vi "FlexMag recipe file.vi"() -> ()   [LabVIEW 2018]
uses:
  <vilib>/Utility/file.llb/Read Delimited Spreadsheet (string).vi
panel:
  in  "redundant":enum32{"Page 1", "Page 2"}(tab)
  in  "dc step length 20":dbl
  in  "dc step length 19":dbl
  in  "dc step length 18":dbl
  in  "dc step length 17":dbl
  in  "dc step length 16":dbl
  in  "dc step length 15":dbl
  in  "dc step length 14":dbl
  in  "dc step length 13":dbl
  in  "dc step length 12":dbl
  in  "dc step length 11":dbl
  in  "dc step length 10":dbl=100.0
  in  "dc step length 9":dbl=100.0
  in  "dc step length 8":dbl=100.0
  in  "dc step length 7":dbl=100.0
  in  "dc step length 6":dbl=100.0
  in  "dc step length 5":dbl=100.0
  in  "dc step length 4":dbl=100.0
  in  "dc step length 3":dbl=100.0
  in  "dc step length 2":dbl=100.0
  in  "dc step length 1":dbl=100.0
  in  "rf step length 20":dbl
  in  "rf step length 19":dbl
  in  "rf step length 18":dbl
  in  "rf step length 17":dbl
  in  "rf step length 16":dbl
  in  "rf step length 15":dbl
  in  "rf step length 14":dbl
  in  "rf step length 13":dbl
  in  "rf step length 12":dbl
  in  "rf step length 11":dbl
  in  "rf step length 1":dbl
  in  "rf step length 2":dbl
  in  "rf step length 3":dbl
  in  "rf step length 4":dbl
  in  "rf step length 5":dbl
  in  "rf step length 6":dbl
  in  "rf step length 7":dbl
  in  "rf step length 8":dbl
  in  "rf step length 9":dbl
  in  "rf step length 10":dbl
  in  "core diameter":dbl=93.0
  in  "left initial diameter":dbl=94.0
  in  "web thickness":dbl=50.0
  out "total length":dbl=500.0
  out "error out 2":errorcluster caption="error out"
  out "error out":errorcluster
  in  "hidden tab":enum32{"Page 1"}(tab)
  out "L dc length step 20":string
  out "L dc length step 19":string
  out "L dc length step 18":string
  out "L dc length step 17":string
  out "L dc length step 16":string
  out "L dc length step 15":string
  out "L dc length step 14":string
  out "L dc length step 13":string
  out "L dc length step 12":string
  out "L dc length step 11":string
  out "L dc power step 20":string
  out "L dc power step 19":string
  out "L dc power step 18":string
  out "L dc power step 17":string
  out "L dc power step 16":string
  out "L dc power step 15":string
  out "L dc power step 14":string
  out "L dc power step 13":string
  out "L dc power step 12":string
  out "L dc power step 11":string
  out "L pressure":string
  out "L argon flow":string
  out "L rf length step 10":string
  out "L rf length step 9":string
  out "L rf length step 8":string
  out "L rf length step 7":string
  out "L rf length step 6":string
  out "L rf length step 5":string
  out "L rf length step 4":string
  out "L rf length step 3":string
  out "L rf length step 2":string
  out "L rf length step 1":string
  out "L rf power step 10":string
  out "L rf power step 9":string
  out "L rf power step 8":string
  out "L rf power step 7":string
  out "L rf power step 6":string
  out "L rf power step 5":string
  out "L rf power step 4":string
  out "L rf power step 3":string
  out "L rf power step 2":string
  out "L rf power step 1":string
  out "L dc length step 10":string
  out "L dc length step 9":string
  out "L dc length step 8":string
  out "L dc length step 7":string
  out "L dc length step 6":string
  out "L dc length step 5":string
  out "L dc length step 4":string
  out "L dc length step 3":string
  out "L dc length step 2":string
  out "L dc length step 1":string
  out "L dc power step 10":string
  out "L dc power step 9":string
  out "L dc power step 8":string
  out "L dc power step 7":string
  out "L dc power step 6":string
  out "L dc power step 5":string
  out "L dc power step 4":string
  out "L dc power step 3":string
  out "L dc power step 2":string
  out "L dc power step 1":string
  out "L microwave power":string
  out "L chamber selection":string
  out "L single process type selection":string
  out "L tension  value":string
  out "L web speed":string
  out "L web thickness":string
  out "L left init diamater":string
  out "L core diamater":string
  out "L web selection":string
  out "L recipe selection":string
  out "L sbs name":string
  out "L recipe name":string
  out "total length error":bool
  out "left diameter after roll":dbl=8.0
  out "done":bool
  out "L dc step number":string
  out "L rf step number":string
  out "L rf length step 11":string
  out "L rf length step 12":string
  out "L rf length step 13":string
  out "L rf length step 14":string
  out "L rf length step 15":string
  out "L rf length step 16":string
  out "L rf length step 17":string
  out "L rf length step 18":string
  out "L rf length step 19":string
  out "L rf length step 20":string
  out "L rf power step 11":string
  out "L rf power step 12":string
  out "L rf power step 13":string
  out "L rf power step 14":string
  out "L rf power step 15":string
  out "L rf power step 16":string
  out "L rf power step 17":string
  out "L rf power step 18":string
  out "L rf power step 19":string
  out "L rf power step 20":string
  in  "steplist tab RF":enum32{"Page 1", "Page 2"}(tab)
  in  "rf step watt 20":dbl
  in  "rf step watt 19":dbl
  in  "rf step watt 18":dbl
  in  "rf step watt 17":dbl
  in  "rf step watt 16":dbl
  in  "rf step watt 15":dbl
  in  "rf step watt 14":dbl
  in  "rf step watt 13":dbl
  in  "rf step watt 12":dbl
  in  "rf step watt 11":dbl
  in  "rf step watt 1":dbl
  in  "rf step watt 2":dbl
  in  "rf step watt 3":dbl
  in  "rf step watt 4":dbl
  in  "rf step watt 7":dbl
  in  "rf step watt 8":dbl
  in  "rf step watt 5":dbl
  in  "rf step watt 6":dbl
  in  "rf step watt 9":dbl
  in  "rf step watt 10":dbl
  in  "Step Number RF":u16(ring) items=["step 1"=1, "step 2"=2, "step 3"=3, "step 4"=4, "step 5"=5, "step 6"=6, "step 7"=7, "step 8"=8, "step 9"=9, "step 10"=10, "step 11"=11, "step 12"=12, "step 13"=13, "step 14"=14, "step 15"=15, "step 16"=16, "step 17"=17, "step 18"=18, "step 19"=19, "step 20"=20]
  out "concatenated string":string
  in  "steplist tab DC":enum32{"Page 1", "Page 2"}(tab)
  in  "dc step watt 1":dbl
  in  "dc step watt 2":dbl
  in  "dc step watt 3":dbl
  in  "dc step watt 4":dbl
  in  "dc step watt 5":dbl
  in  "dc step watt 6":dbl
  in  "dc step watt 7":dbl
  in  "dc step watt 8":dbl
  in  "dc step watt 9":dbl
  in  "dc step watt 10":dbl
  in  "Step Number DC":u16(ring) items=["step 1"=1, "step 2"=2, "step 3"=3, "step 4"=4, "step 5"=5, "step 6"=6, "step 7"=7, "step 8"=8, "step 9"=9, "step 10"=10, "step 11"=11, "step 12"=12, "step 13"=13, "step 14"=14, "step 15"=15, "step 16"=16, "step 17"=17, "step 18"=18, "step 19"=19, "step 20"=20]
  in  "dc step watt 20":dbl
  in  "dc step watt 19":dbl
  in  "dc step watt 18":dbl
  in  "dc step watt 17":dbl
  in  "dc step watt 16":dbl
  in  "dc step watt 15":dbl
  in  "dc step watt 14":dbl
  in  "dc step watt 13":dbl
  in  "dc step watt 12":dbl
  in  "dc step watt 11":dbl
  in  "General tab sub vi":enum32{"Page 1"}(tab)
  in  "Pressure set mbar":dbl=0.007 format="%#_1e"
  in  "Ar set sccm":dbl=40.0
  in  "CANCEL":bool
  in  "SAVE":bool
  in  "web-other tab":T1(tab)
  in  "tension value":dbl=10.0
  in  "web speed":dbl=550.0
  in  "CALCULATE":bool
  in  "Web Selection":u16(ring) items=["web", "other"]
  in  "Recipe Selection":u16(ring) items=["single recipe", "multilayer recipe"]
  in  "Recipe Name":string
  in  "Substrate Material":string
  in  "recipe selection":T2(tab)
  in  "single process selection":enum32{"microwave", "dcsputter", "rfsputter"}(radio)
  in  "single process selection":T3(tab)
  in  "power microwave":dbl
  in  "DC Sputter Chamber Selection":enum32{"chamber II", "chamber III"}(radio)
  in  "power rf":dbl
  in  "web speed ch III ml":dbl=250.0
  in  "web speed ch II ml":dbl=250.0
  in  "LOAD":bool
  in  "SHOW":bool
  in  "password":string
  # "length(cm)"
  # "length(cm)"
  # "Core Diameter"
  # "mm"
  # "Left InitialDiameter"
  # "mm"
  # "µm"
  # "Web Thickness"
  # "cm"
  # "Total Length"
  # "Step List(RF)"
  # "Step Number"
  # "power(watt)"
  # "Step 1"
  # "Step 2"
  # "Step 3"
  # "Step 4"
  # "Step 5"
  # "Step 6"
  # "Step 7"
  # "Step 8"
  # "Step 9"
  # "Step 10"
  # "Step 11"
  # "Step 12"
  # "Step 13"
  # "Step 14"
  # "Step 15"
  # "Step 16"
  # "Step 17"
  # "Step 18"
  # "Step 19"
  # "Step 20"
  # "Step List(DC)"
  # "Stem Number"
  # "power(watt)"
  # "Step 1"
  # "Step 2"
  # "Step 3"
  # "Step 4"
  # "Step 5"
  # "Step 6"
  # "Step 7"
  # "Step 8"
  # "Step 9"
  # "Step 10"
  # "Step 11"
  # "Step 12"
  # "Step 13"
  # "Step 14"
  # "Step 15"
  # "Step 16"
  # "Step 17"
  # "Step 18"
  # "Step 19"
  # "Step 20"
  # "Recipe Name"
  # "Subsrate Material"
  # "Recipe Selection"
  # "Web Selection"
  # "Argon Flow"
  # "sccm"
  # "Set Pressure"
  # "mbar"
  # "Web Speed"
  # "cm/min"
  # "Tension Value"
  # "N"
  # "Power"
  # "watt"
  # "Power"
  # "watt"
  # "DCPS PARAMETERS"
  # "Chamber III"
  # "Chamber II"
  # "Web Speed"
  # "cm/min"
  # "Web Speed"
  # "cm/min"
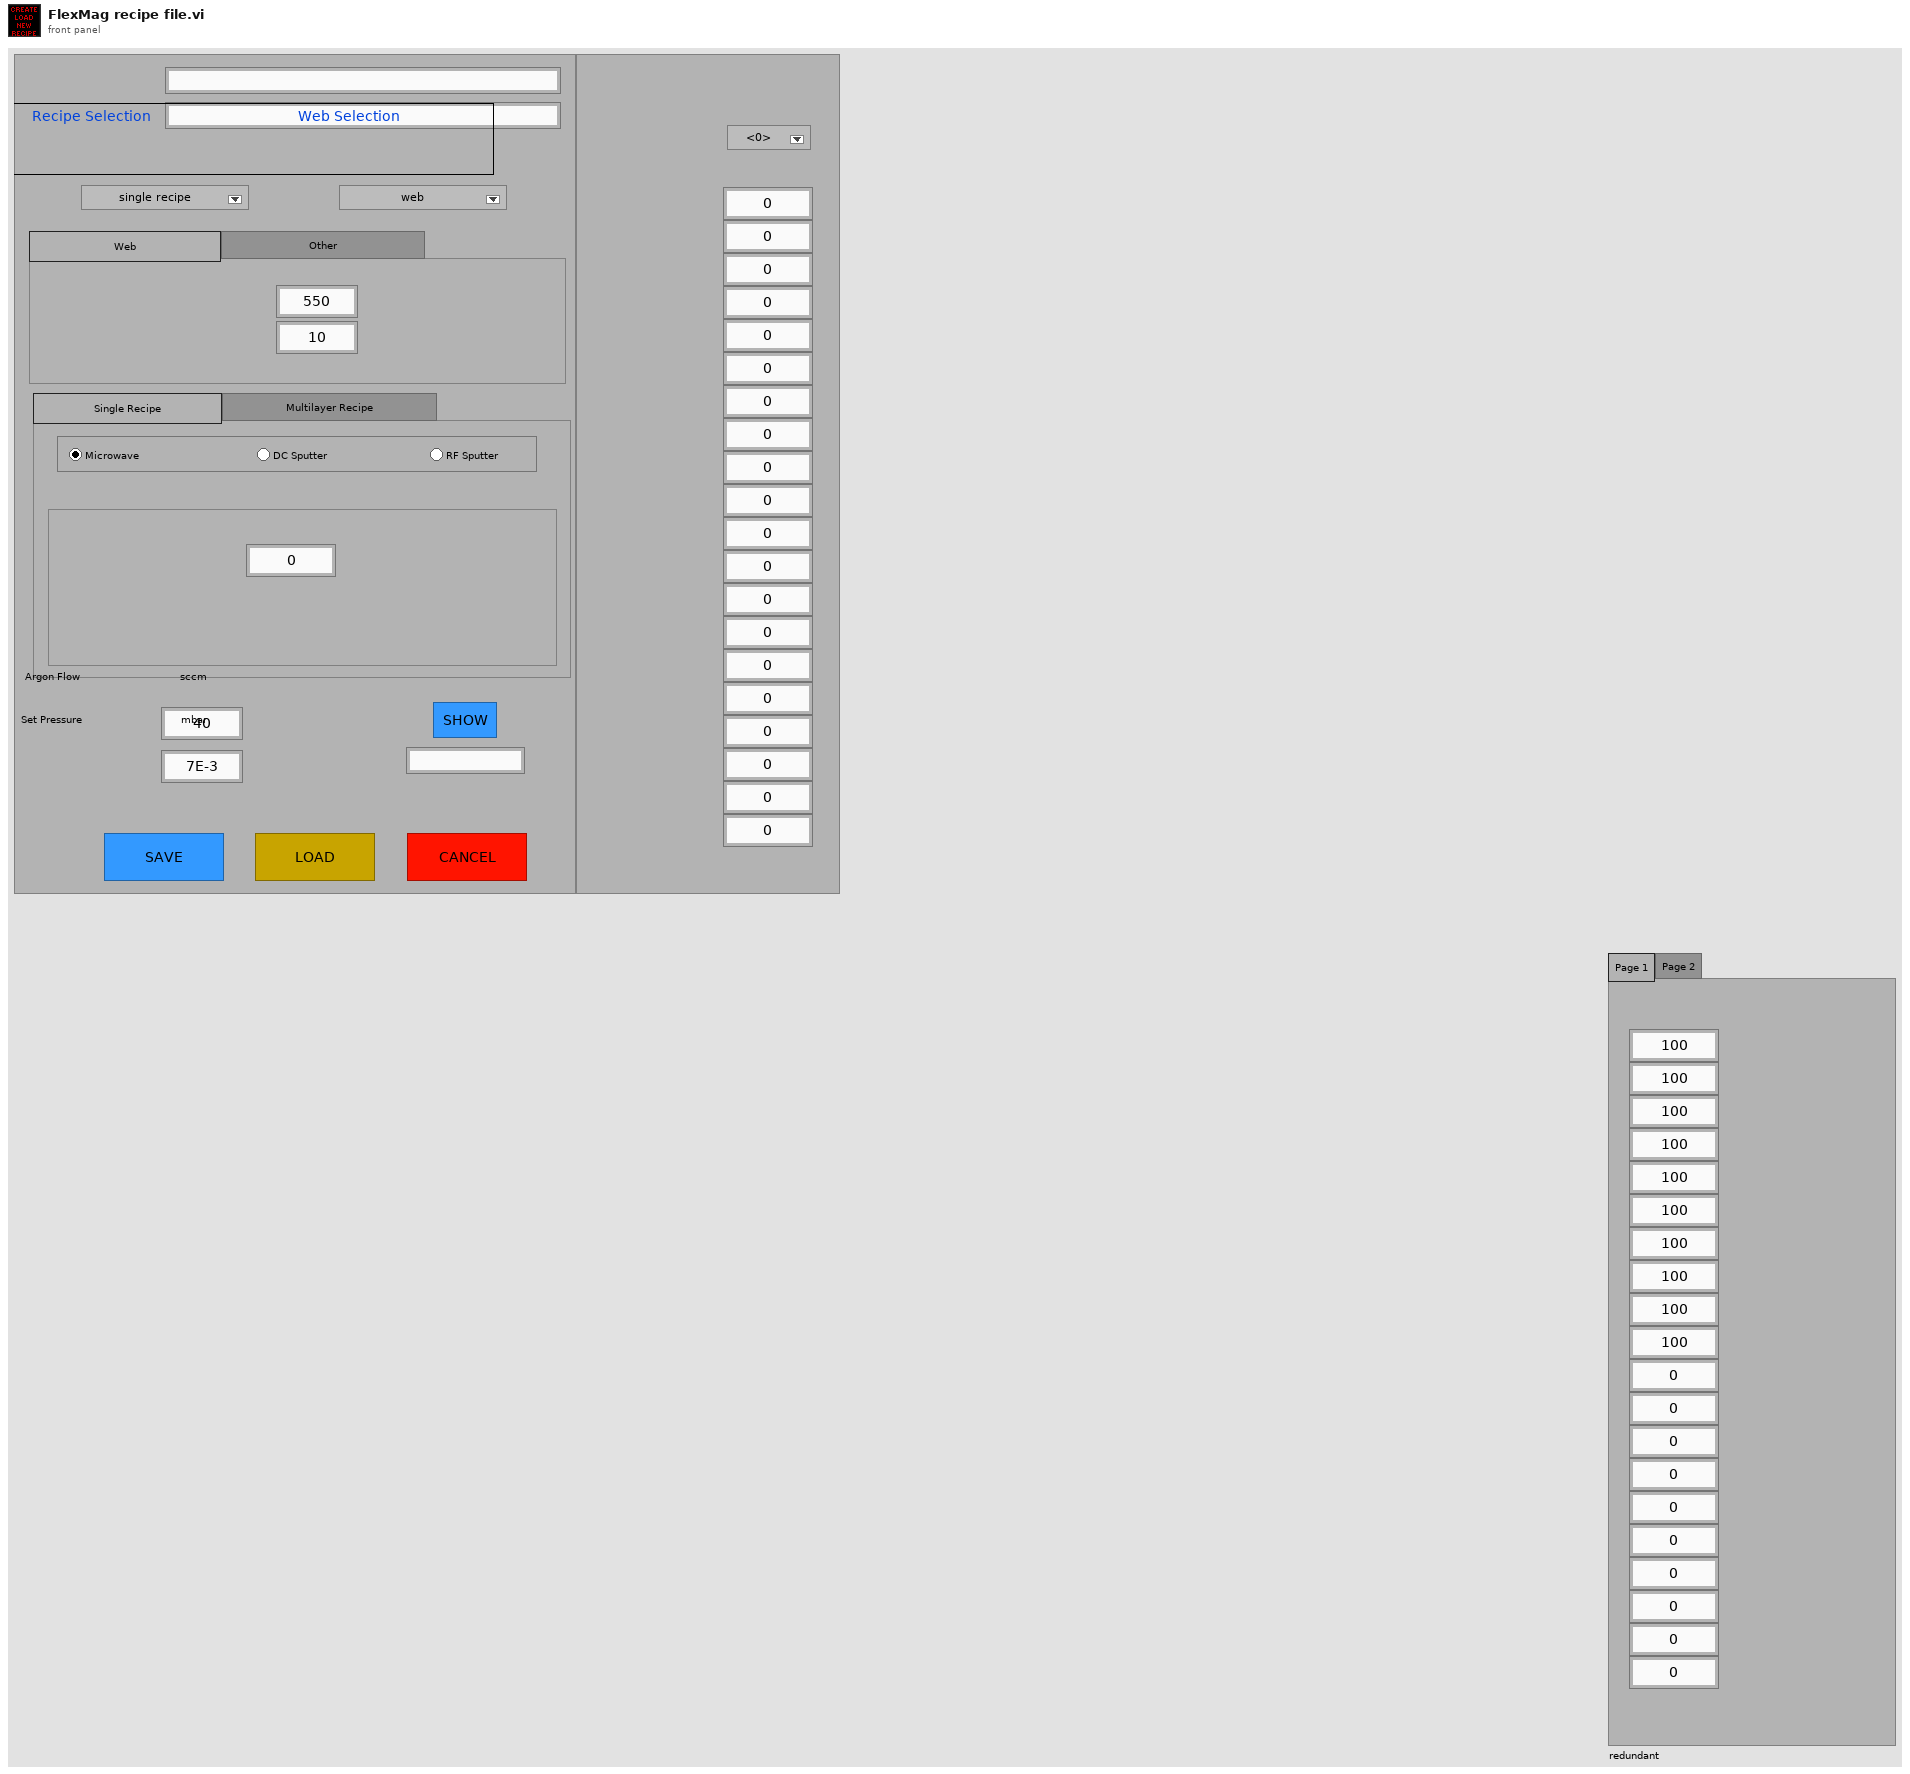
[diagram p1: front panel]
types:
  T1 = enum32{"Web                                                    ", "Other                                                      "}
  T2 = enum32{"Single Recipe                                    ", "Multilayer Recipe                                      "}
  T3 = enum32{"Microwave                ", "DC Sputter                   ", "RF Sputter                         "}
  T4 = enum16{"open", "replace", "create", "open or create", "replace or create", "replace or create with confirmation"}
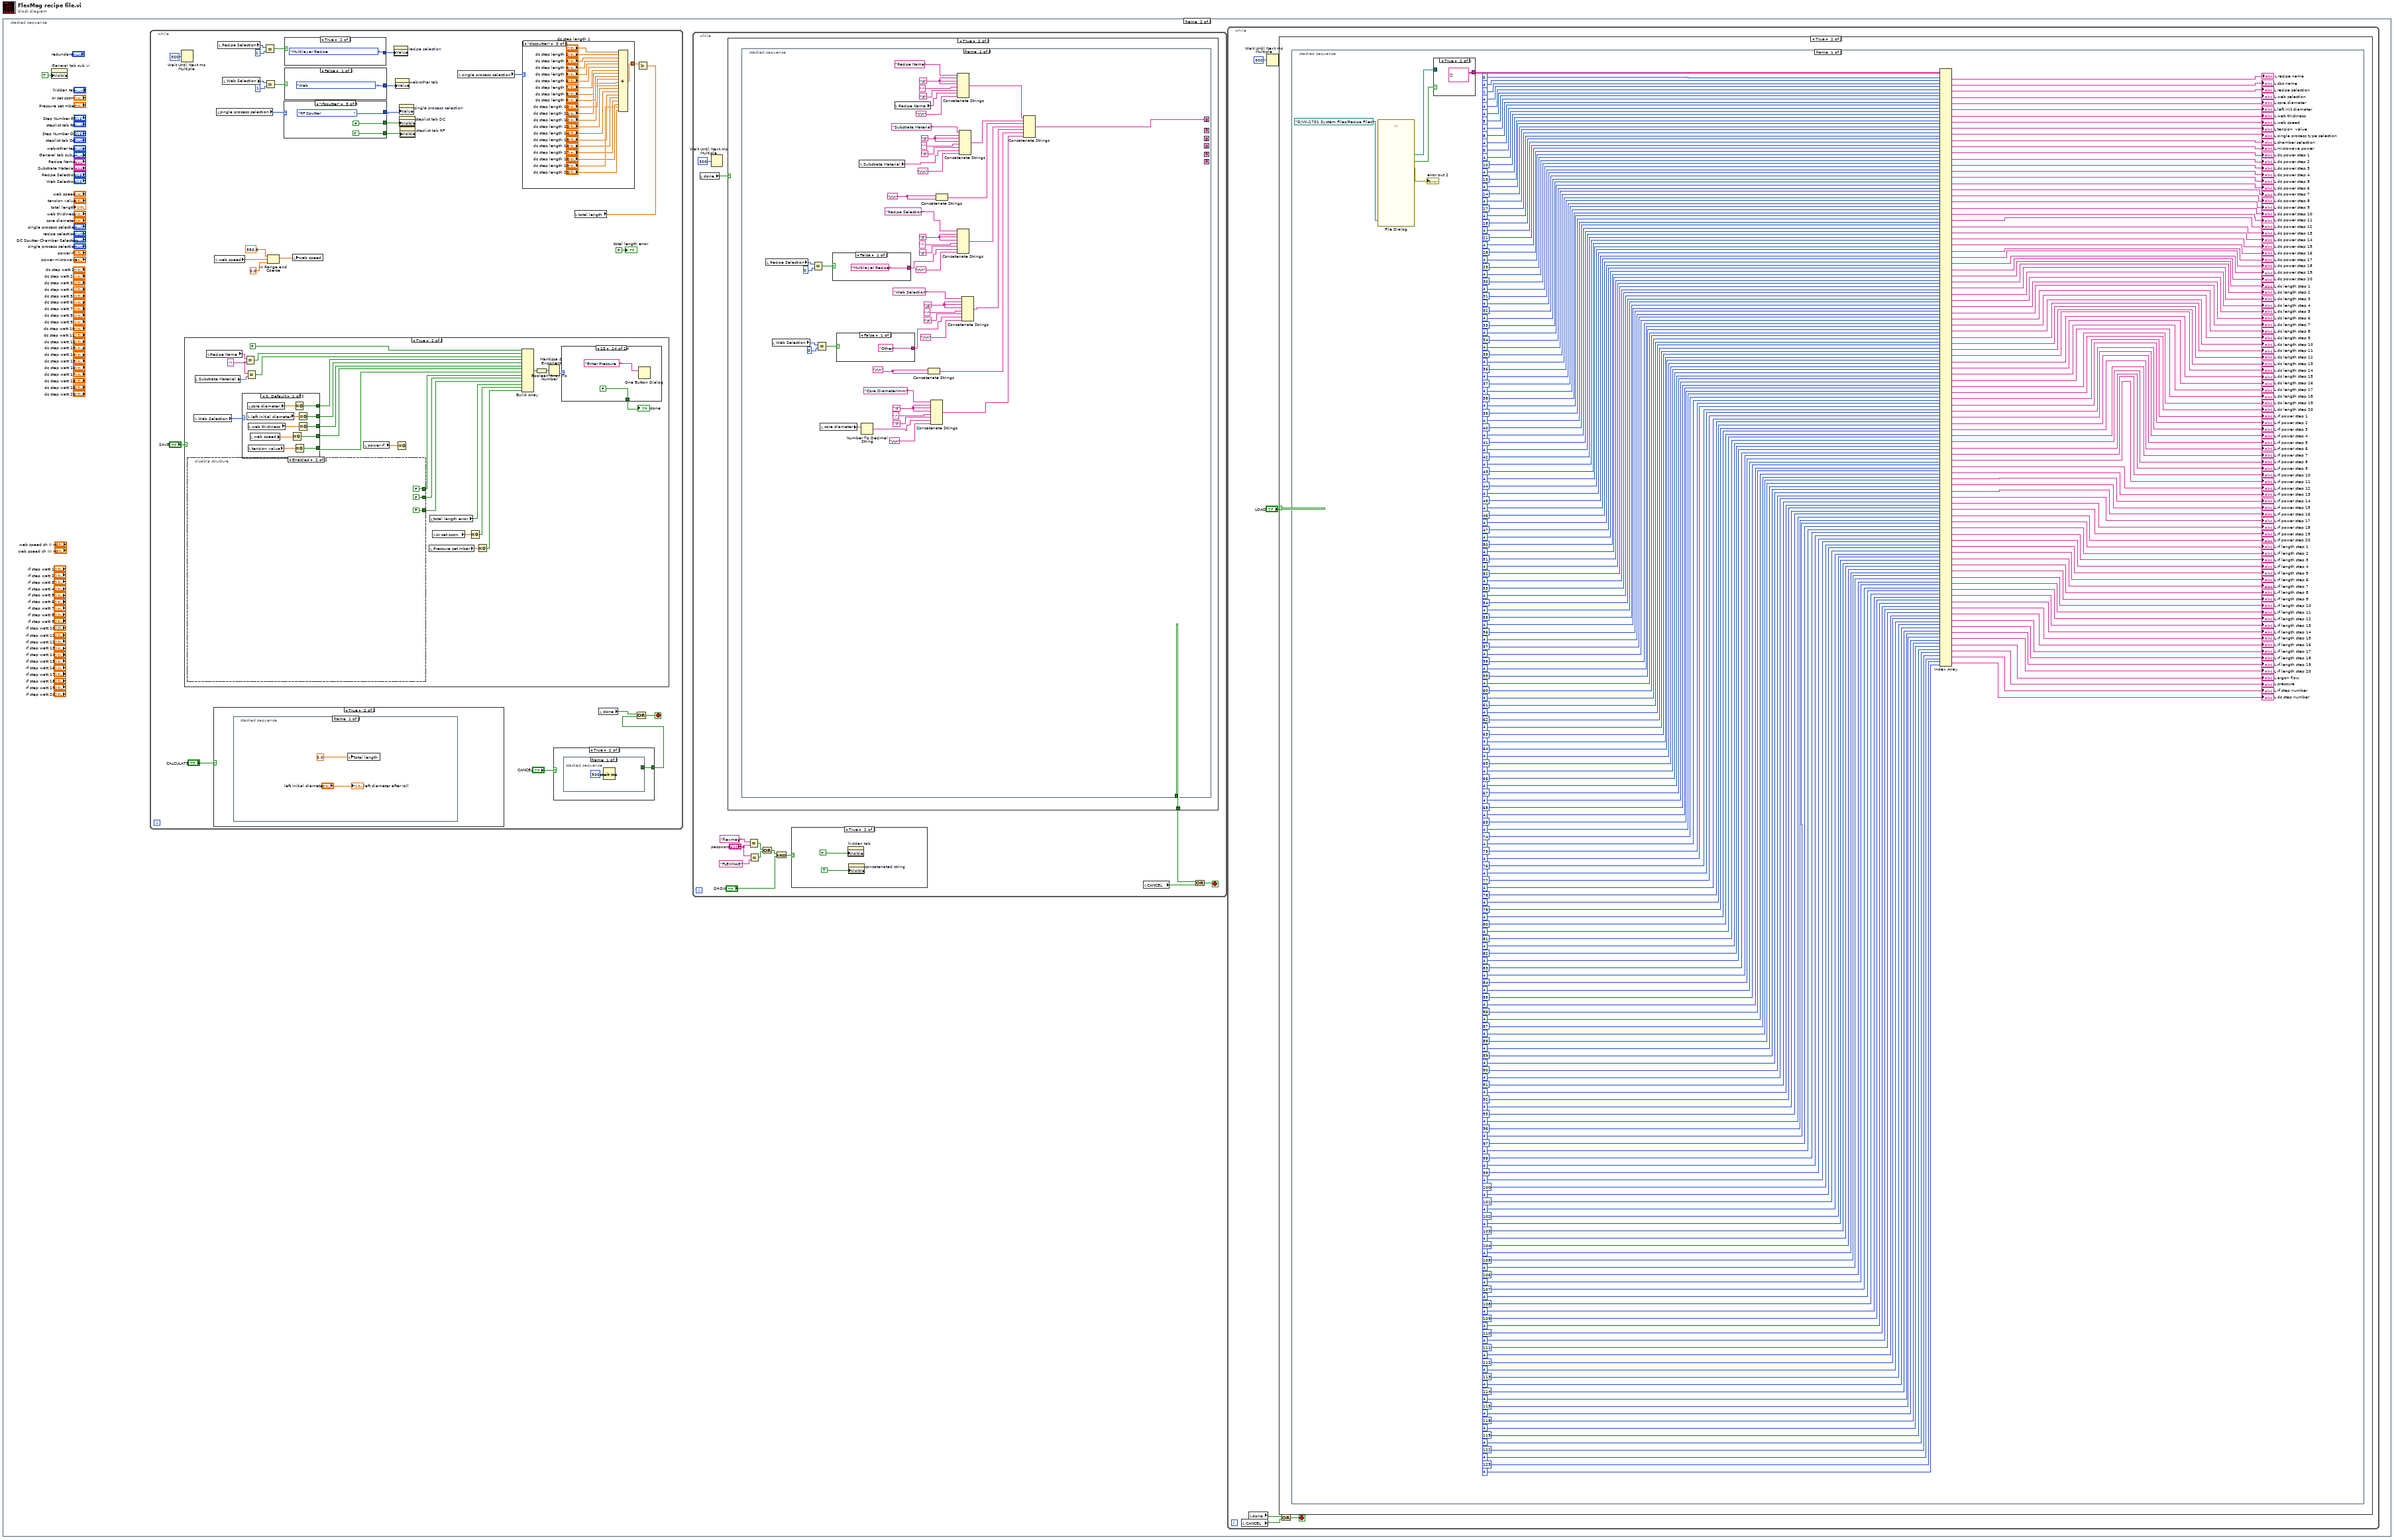
[diagram p0: block diagram]
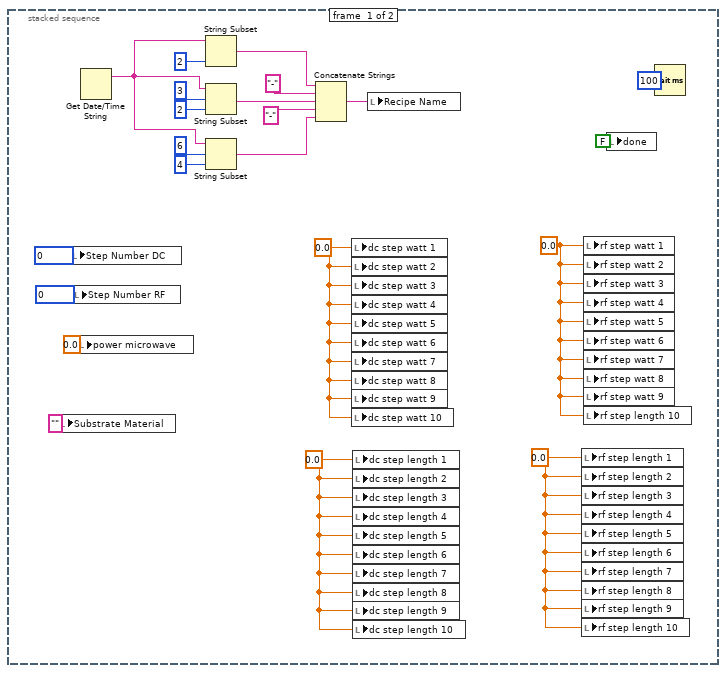
[diagram p2: hidden frame]
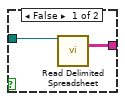
[diagram p4: hidden frame]
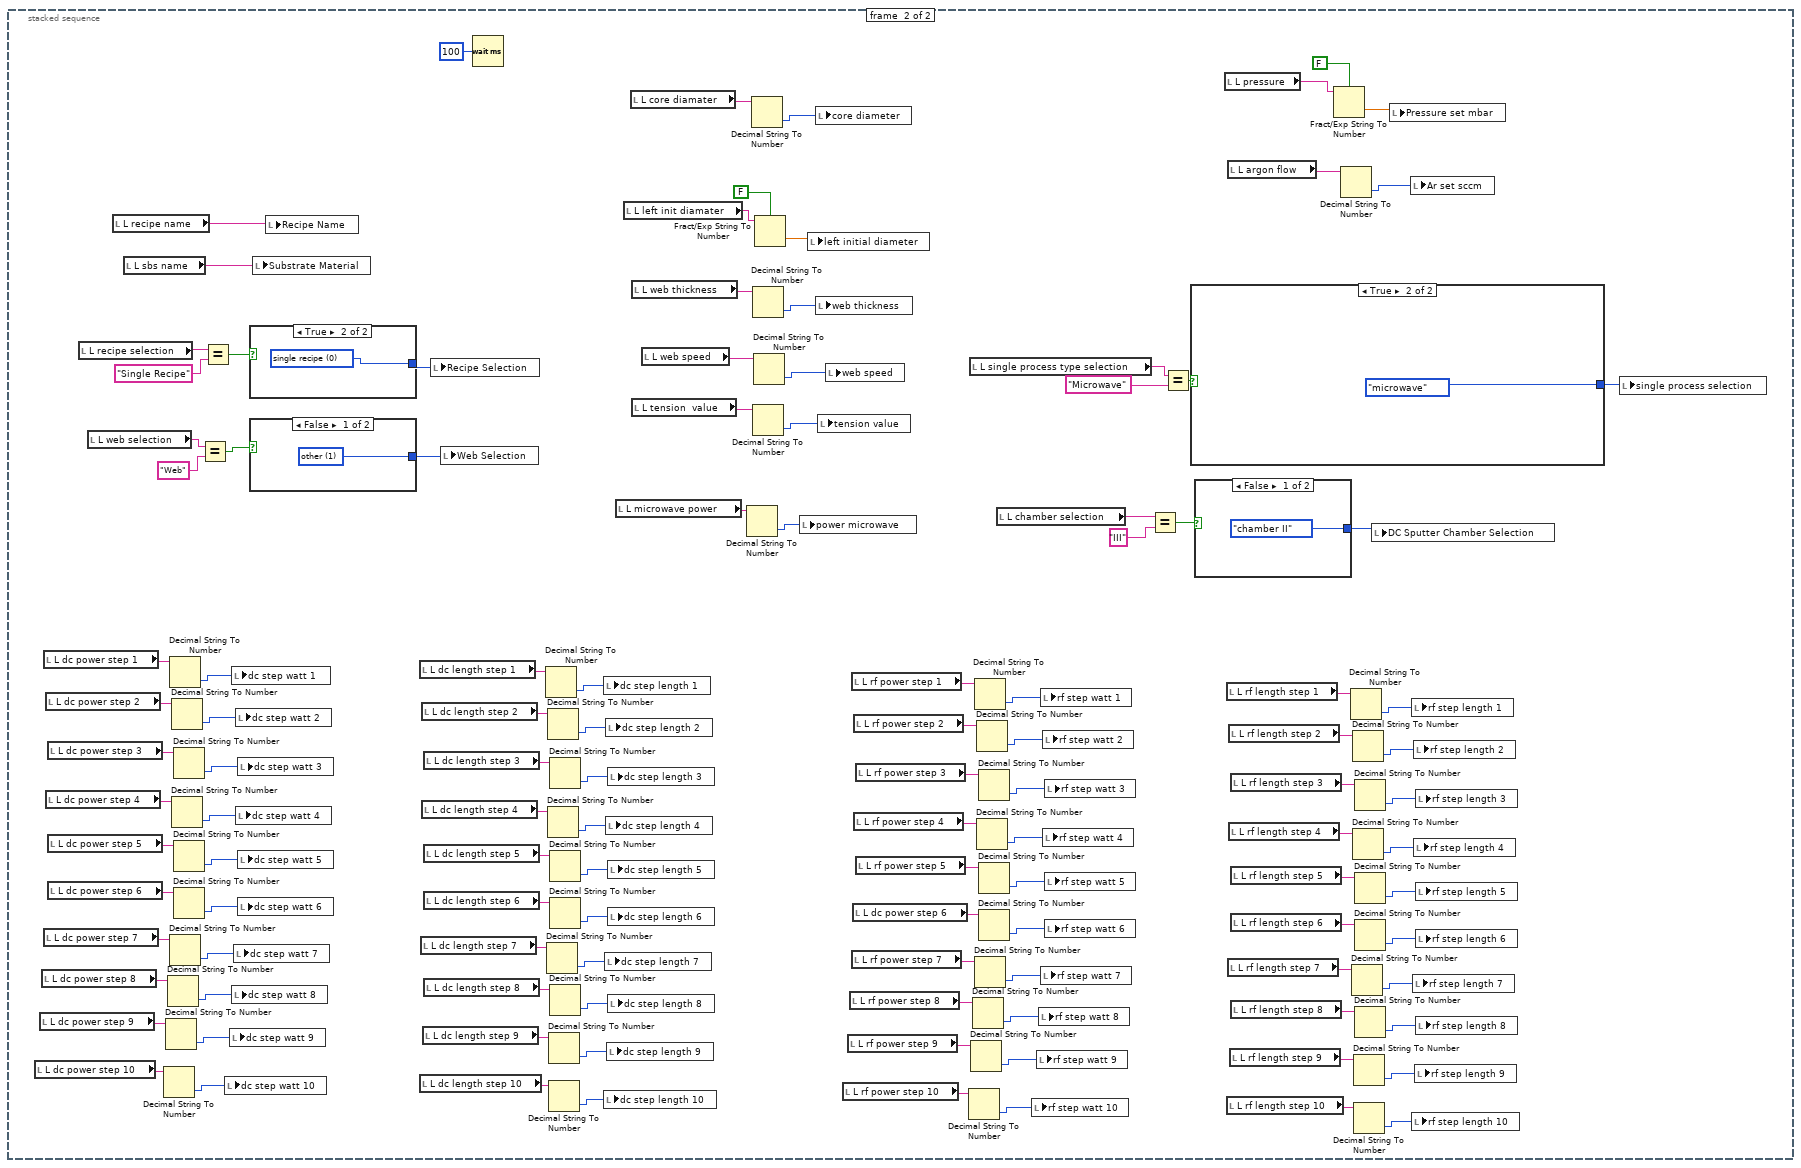
[diagram p5: hidden frame]
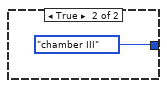
[diagram p6: hidden frame]
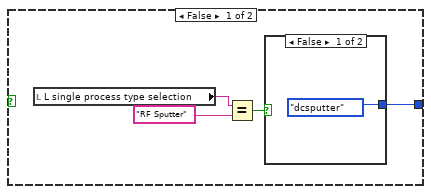
[diagram p7: hidden frame]
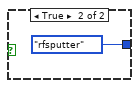
[diagram p8: hidden frame]
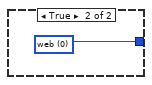
[diagram p9: hidden frame]
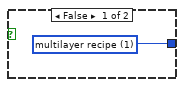
[diagram p10: hidden frame]
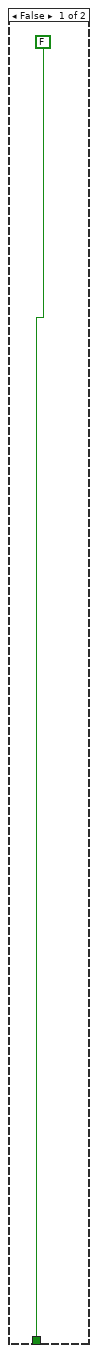
[diagram p12: hidden frame]
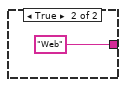
[diagram p13: hidden frame]
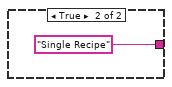
[diagram p14: hidden frame]
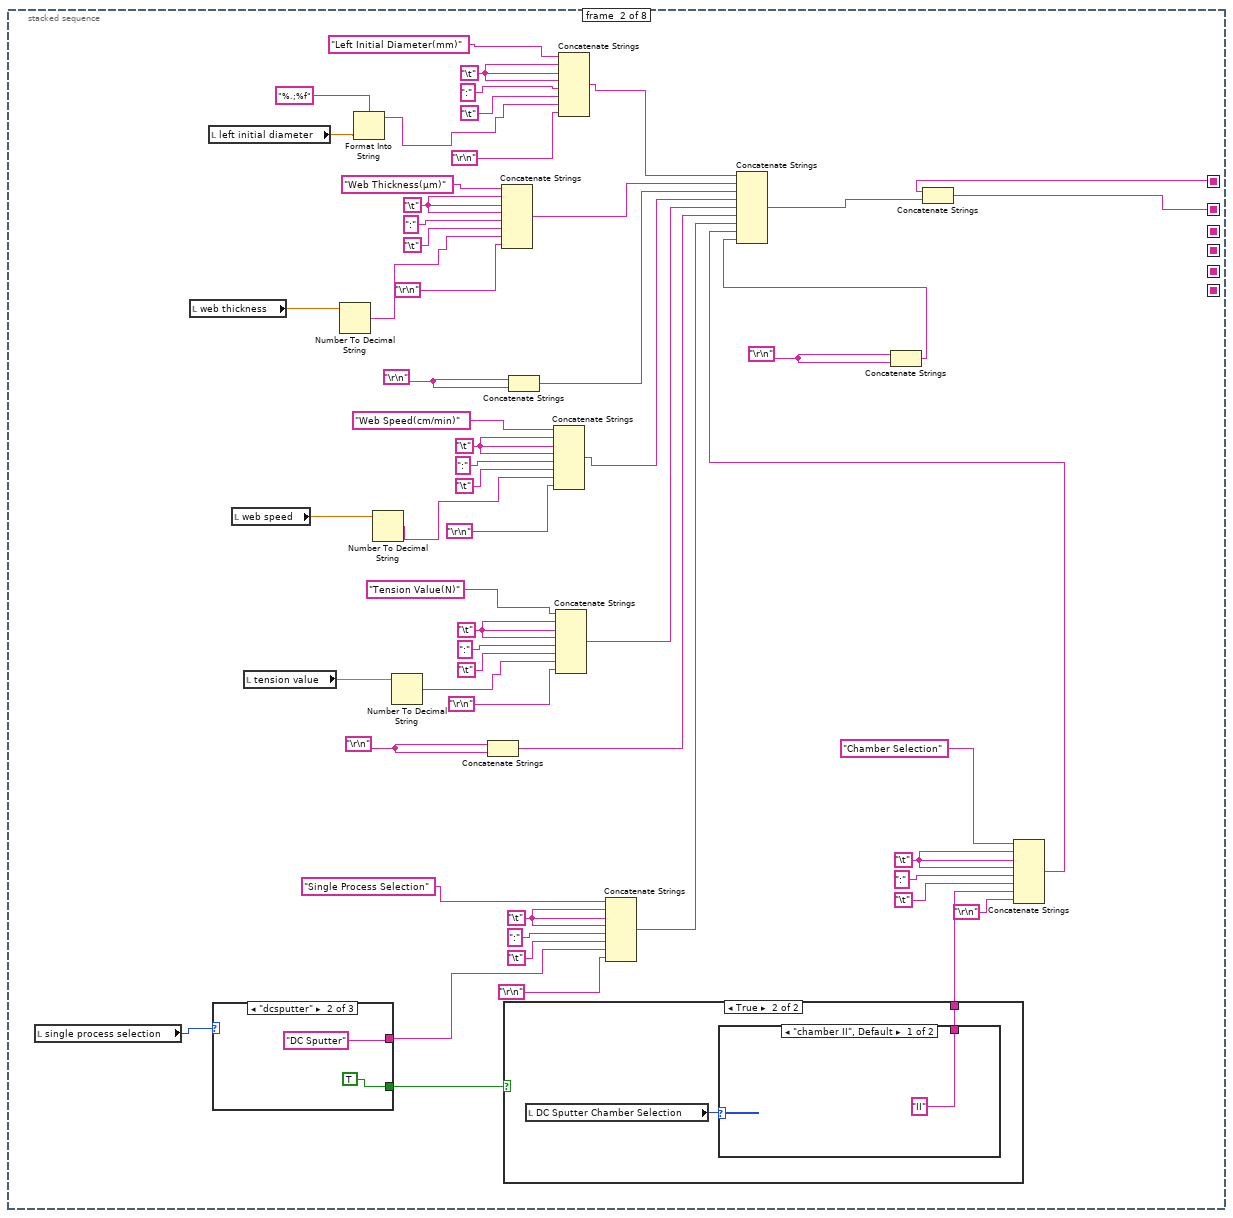
[diagram p15: hidden frame]
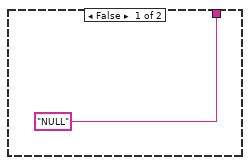
[diagram p16: hidden frame]
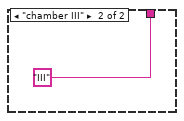
[diagram p17: hidden frame]
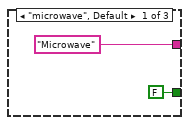
[diagram p18: hidden frame]
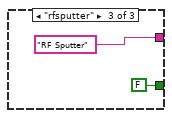
[diagram p19: hidden frame]
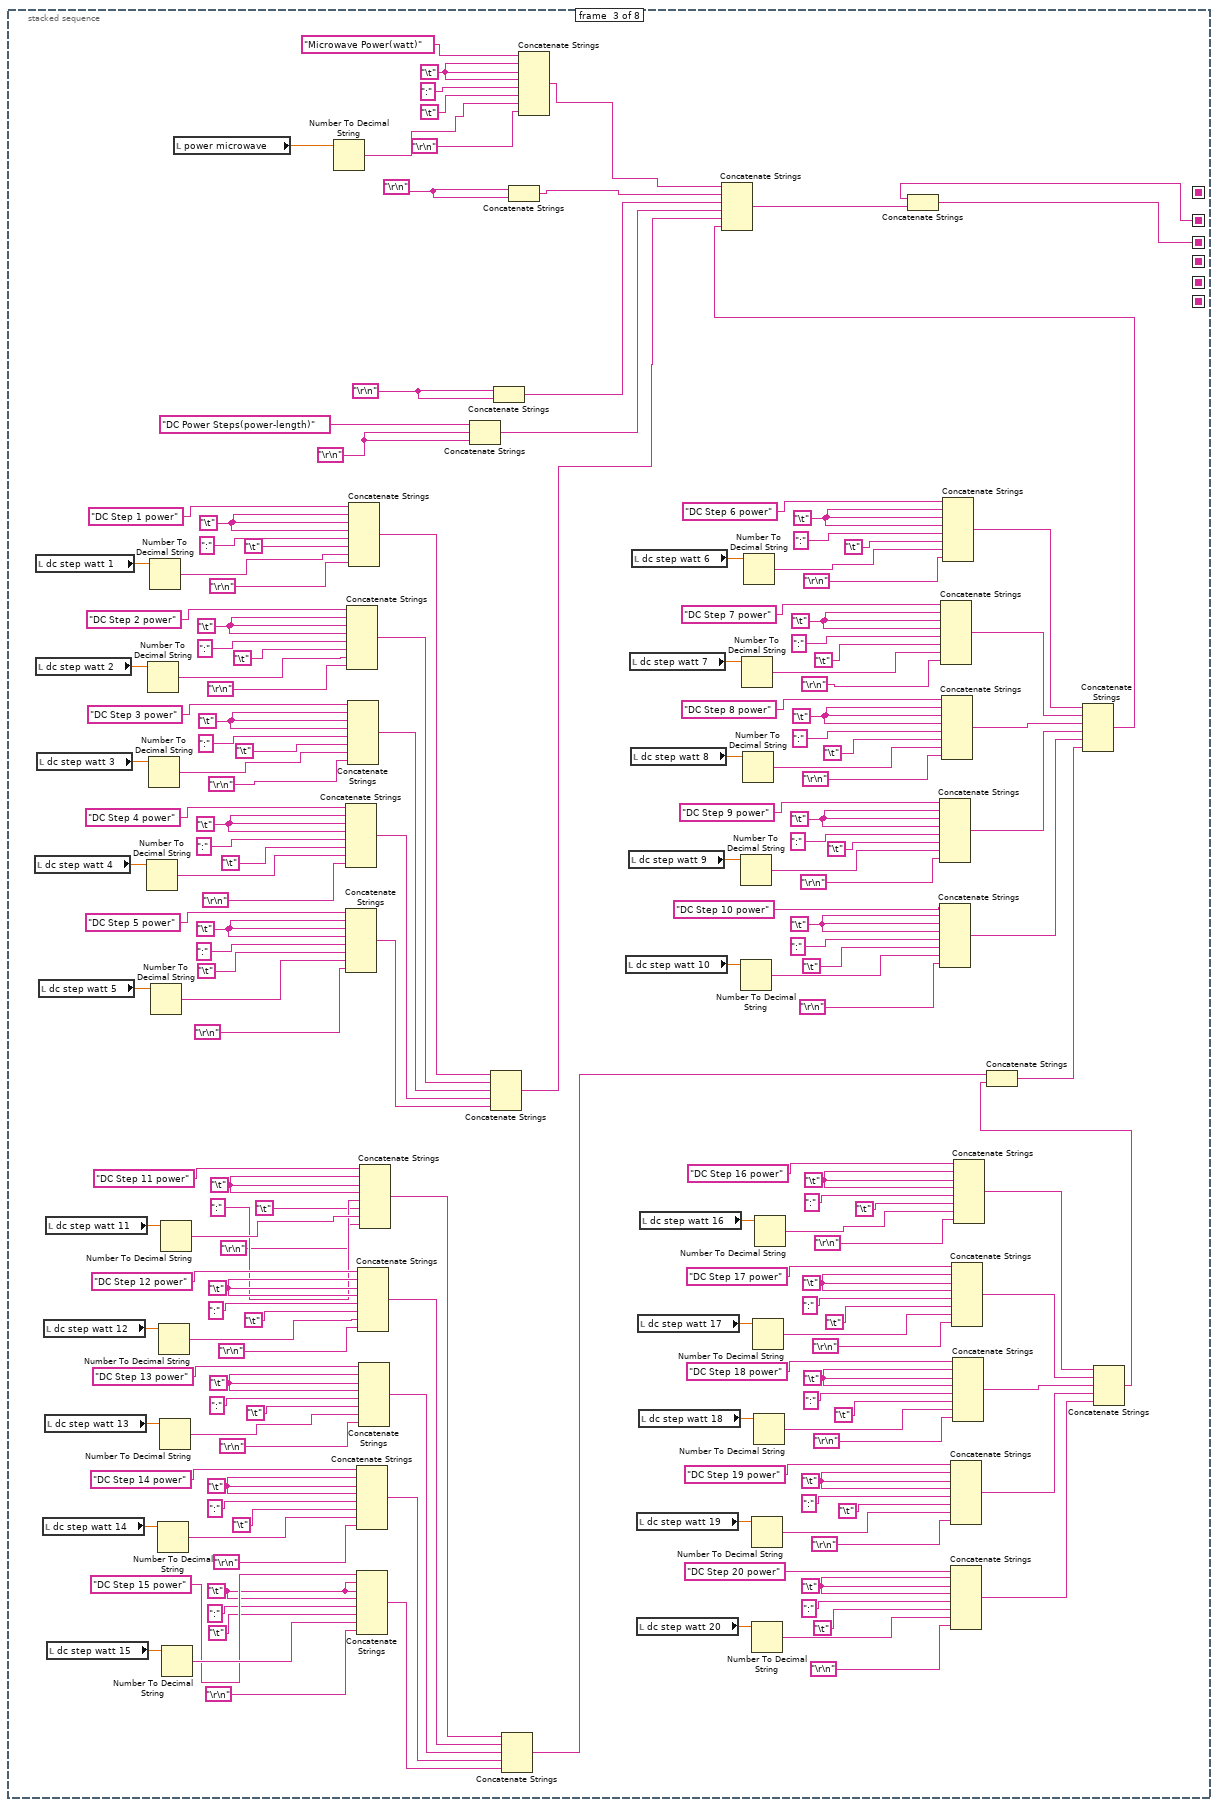
[diagram p20: hidden frame]
diagram:
  n1 = stacked-sequence {
    frame #0 {
      w3 = u16 0 items=["step 1"=1, "step 2"=2, "step 3"=3, "step 4"=4, "step 5"=5, "step 6"=6, "step 7"=7, "step 8"=8, "step 9"=9, "step 10"=10] ("Step Number DC")
      w5 = 0.0 ("dc step watt 1")
      w4 = 0.0 ("dc step watt 1")
      w6 = u16 0 items=["step 1"=1, "step 2"=2, "step 3"=3, "step 4"=4, "step 5"=5, "step 6"=6, "step 7"=7, "step 8"=8, "step 9"=9, "step 10"=10] ("Step Number DC")
      w7 = 0.0 ("dc step watt 1")
      w8 = 0.0 ("dc step watt 1")
      n2 = local write "Substrate Material"("" ("Substrate Material")) -> ()
      n3 = local write "Step Number DC"(w6) -> ()
      n4 = local write "Step Number RF"(w3) -> ()
      n5 = local write "power microwave"(0.0 ("power microwave")) -> ()
      n6 = Get Date/Time String() -> (date string=w16:string)  [unwired: 3 in, 1 out]
      n7 = String Subset(string=w16, length (rest)=2 ("length (rest)")) -> (substring=w17:string)  [unwired: 1 in]
      n8 = String Subset(string=w16, offset (0)=3, length (rest)=2 ("length (rest)")) -> (substring=w18:string)
      n9 = String Subset(string=w16, offset (0)=6, length (rest)=4 ("length (rest)")) -> (substring=w19:string)
      n10 = Concatenate Strings(w17, "-" ("string"), w18, "-" ("string"), w19) -> (w20:string)
      n11 = local write "dc step watt 1"(w8) -> ()
      n12 = local write "dc step watt 2"(w8) -> ()
      n13 = local write "dc step watt 3"(w8) -> ()
      n14 = local write "dc step watt 4"(w8) -> ()
      n15 = local write "dc step watt 5"(w8) -> ()
      n16 = local write "dc step watt 6"(w8) -> ()
      n17 = local write "dc step watt 7"(w8) -> ()
      n18 = local write "dc step watt 8"(w8) -> ()
      n19 = local write "dc step watt 9"(w8) -> ()
      n20 = local write "dc step watt 10"(w8) -> ()
      n21 = local write "dc step length 1"(w7) -> ()
      n22 = local write "dc step length 2"(w7) -> ()
      n23 = local write "dc step length 3"(w7) -> ()
      n24 = local write "dc step length 4"(w7) -> ()
      n25 = local write "dc step length 5"(w7) -> ()
      n26 = local write "dc step length 6"(w7) -> ()
      n27 = local write "dc step length 7"(w7) -> ()
      n28 = local write "dc step length 8"(w7) -> ()
      n29 = local write "dc step length 9"(w7) -> ()
      n30 = local write "dc step length 10"(w7) -> ()
      n31 = local write "Recipe Name"(w20) -> ()
      n32 = local write "rf step length 1"(w5) -> ()
      n33 = local write "rf step length 2"(w5) -> ()
      n34 = local write "rf step length 3"(w5) -> ()
      n35 = local write "rf step length 4"(w5) -> ()
      n36 = local write "rf step length 5"(w5) -> ()
      n37 = local write "rf step length 6"(w5) -> ()
      n38 = local write "rf step length 7"(w5) -> ()
      n39 = local write "rf step length 8"(w5) -> ()
      n40 = local write "rf step length 9"(w5) -> ()
      n41 = local write "rf step length 10"(w5) -> ()
      n42 = local write "rf step watt 1"(w4) -> ()
      n43 = local write "rf step watt 2"(w4) -> ()
      n44 = local write "rf step watt 3"(w4) -> ()
      n45 = local write "rf step watt 4"(w4) -> ()
      n46 = local write "rf step watt 5"(w4) -> ()
      n47 = local write "rf step watt 6"(w4) -> ()
      n48 = local write "rf step watt 7"(w4) -> ()
      n49 = local write "rf step watt 8"(w4) -> ()
      n50 = local write "rf step watt 9"(w4) -> ()
      n51 = local write "rf step length 10"(w4) -> ()
      n52 = local write "done"(FALSE ("done")) -> ()
      n53 = Wait (ms)(milliseconds to wait=u32 100) -> ()  [unwired: 1 out]
    }
    frame #1 {
      n54 = property on="General tab sub vi" class="TabCtl (strict)"("Visible"=TRUE) -> ()  [unwired: 2 in, 2 out]
      n55 = while {
        stop <- w1354 stop-if-true
        n56 = Wait Until Next ms Multiple(millisecond multiple=u32 300) -> ()  [unwired: 1 out]
        n57 = case shown="True" "SAVE" {
          frame False {
          }
          frame True {
            w1468 = "" ("y")
            n58 = disable-structure shown="Enabled" {
              disable-tunnel: [w1474 FALSE] -> w1455
              disable-tunnel: [w1473 FALSE] -> w1454
              disable-tunnel: [w1472 FALSE] -> w1453
              frame Disabled {
                n59 = local read "single process selection"() -> (w1476:enum32{"microwave", "dcsputter", "rfsputter"})
                n60 = local read "Recipe Selection"() -> (w1477:u16)
                n61 = local read "Step Number DC"() -> (w1475:u16)
                n62 = local read "Step Number RF"() -> (w1471:u16)
                n63 = case shown="0, Default" w1477 {
                  tunnel: w1476 -> [w1483 _]
                  tunnel: w1475 -> [w1482 _]
                  tunnel: [w1481 FALSE] -> w1474
                  tunnel: [w1480 FALSE] -> w1473
                  tunnel: [w1479 FALSE] -> w1472
                  tunnel: w1471 -> [w1478 _]
                  frame 0, Default {
                    # "single recipe"
                    n64 = case shown="\"dcsputter\"" w1483 {
                      tunnel: w1482 -> [_ w1491 _]
                      tunnel: [w1486 FALSE FALSE] -> w1481
                      tunnel: [FALSE w1490 FALSE] -> w1480
                      tunnel: [FALSE FALSE w1724] -> w1479
                      tunnel: w1478 -> [_ _ w1723]
                      frame "microwave", Default {
                        n65 = local read "power microwave"() -> (w1487:dbl)
                        n66 = Equal To 0?(x=w1487) -> (x = 0?=w1486:bool)
                      }
                      frame "dcsputter" {
                        n67 = case shown="1" w1491 {
                          tunnel: [FALSE w1493 w1502 w1515 w1532 w1553 w1578 w1607 w1640 w1677 w1718] -> w1490
                          frame 0, Default {
                          }
                          frame 1 {
                            n68 = local read "dc step length 1"() -> (w1496:dbl)
                            n69 = local read "dc step watt 1"() -> (w1497:dbl)
                            n70 = Equal To 0?(x=w1497) -> (x = 0?=w1495:bool)
                            n71 = Equal To 0?(x=w1496) -> (x = 0?=w1494:bool)
                            n72 = Compound Arithmetic op=OR(w1495, w1494) -> (w1493:bool)
                          }
                          frame 2 {
                            n73 = local read "dc step length 1"() -> (w1505:dbl)
                            n74 = local read "dc step length 2"() -> (w1501:dbl)
                            n75 = local read "dc step watt 1"() -> (w1506:dbl)
                            n76 = local read "dc step watt 2"() -> (w1500:dbl)
                            n77 = Equal To 0?(x=w1506) -> (x = 0?=w1504:bool)
                            n78 = Equal To 0?(x=w1500) -> (x = 0?=w1499:bool)
                            n79 = Equal To 0?(x=w1505) -> (x = 0?=w1503:bool)
                            n80 = Equal To 0?(x=w1501) -> (x = 0?=w1498:bool)
                            n81 = Compound Arithmetic op=OR(w1504, w1503, w1499, w1498) -> (w1502:bool)
                          }
                          frame 3 {
                            n82 = local read "dc step length 1"() -> (w1518:dbl)
                            n83 = local read "dc step length 2"() -> (w1514:dbl)
                            n84 = local read "dc step length 3"() -> (w1509:dbl)
                            n85 = local read "dc step watt 1"() -> (w1519:dbl)
                            n86 = local read "dc step watt 2"() -> (w1513:dbl)
                            n87 = local read "dc step watt 3"() -> (w1510:dbl)
                            n88 = Equal To 0?(x=w1519) -> (x = 0?=w1517:bool)
                            n89 = Equal To 0?(x=w1513) -> (x = 0?=w1512:bool)
                            n90 = Equal To 0?(x=w1518) -> (x = 0?=w1516:bool)
                            n91 = Equal To 0?(x=w1510) -> (x = 0?=w1508:bool)
                            n92 = Equal To 0?(x=w1514) -> (x = 0?=w1511:bool)
                            n93 = Equal To 0?(x=w1509) -> (x = 0?=w1507:bool)
                            n94 = Compound Arithmetic op=OR(w1517, w1516, w1512, w1511, w1508, w1507) -> (w1515:bool)
                          }
                          frame 4 {
                            n95 = local read "dc step length 1"() -> (w1535:dbl)
                            n96 = local read "dc step length 4"() -> (w1523:dbl)
                            n97 = local read "dc step length 2"() -> (w1531:dbl)
                            n98 = local read "dc step length 3"() -> (w1526:dbl)
                            n99 = local read "dc step watt 1"() -> (w1536:dbl)
                            n100 = local read "dc step watt 2"() -> (w1530:dbl)
                            n101 = local read "dc step watt 4"() -> (w1522:dbl)
                            n102 = local read "dc step watt 3"() -> (w1527:dbl)
                            n103 = Equal To 0?(x=w1536) -> (x = 0?=w1534:bool)
                            n104 = Equal To 0?(x=w1530) -> (x = 0?=w1529:bool)
                            n105 = Equal To 0?(x=w1522) -> (x = 0?=w1521:bool)
                            n106 = Equal To 0?(x=w1535) -> (x = 0?=w1533:bool)
                            n107 = Equal To 0?(x=w1527) -> (x = 0?=w1525:bool)
                            n108 = Equal To 0?(x=w1523) -> (x = 0?=w1520:bool)
                            n109 = Equal To 0?(x=w1531) -> (x = 0?=w1528:bool)
                            n110 = Equal To 0?(x=w1526) -> (x = 0?=w1524:bool)
                            n111 = Compound Arithmetic op=OR(w1534, w1533, w1529, w1528, w1525, w1524, w1521, w1520) -> (w1532:bool)
                          }
                          frame 5 {
                            n112 = local read "dc step length 5"() -> (w1539:dbl)
                            n113 = local read "dc step length 1"() -> (w1556:dbl)
                            n114 = local read "dc step length 4"() -> (w1544:dbl)
                            n115 = local read "dc step length 2"() -> (w1552:dbl)
                            n116 = local read "dc step length 3"() -> (w1547:dbl)
                            n117 = local read "dc step watt 1"() -> (w1557:dbl)
                            n118 = local read "dc step watt 5"() -> (w1540:dbl)
                            n119 = local read "dc step watt 2"() -> (w1551:dbl)
                            n120 = local read "dc step watt 4"() -> (w1543:dbl)
                            n121 = local read "dc step watt 3"() -> (w1548:dbl)
                            n122 = Equal To 0?(x=w1540) -> (x = 0?=w1538:bool)
                            n123 = Equal To 0?(x=w1557) -> (x = 0?=w1555:bool)
                            n124 = Equal To 0?(x=w1539) -> (x = 0?=w1537:bool)
                            n125 = Equal To 0?(x=w1551) -> (x = 0?=w1550:bool)
                            n126 = Equal To 0?(x=w1543) -> (x = 0?=w1542:bool)
                            n127 = Equal To 0?(x=w1556) -> (x = 0?=w1554:bool)
                            n128 = Equal To 0?(x=w1548) -> (x = 0?=w1546:bool)
                            n129 = Equal To 0?(x=w1544) -> (x = 0?=w1541:bool)
                            n130 = Equal To 0?(x=w1552) -> (x = 0?=w1549:bool)
                            n131 = Equal To 0?(x=w1547) -> (x = 0?=w1545:bool)
                            n132 = Compound Arithmetic op=OR(w1555, w1554, w1550, w1549, w1546, w1545, w1542, w1541, w1538, w1537) -> (w1553:bool)
                          }
                          frame 6 {
                            n133 = local read "dc step length 6"() -> (w1561:dbl)
                            n134 = local read "dc step length 5"() -> (w1564:dbl)
                            n135 = local read "dc step length 1"() -> (w1581:dbl)
                            n136 = local read "dc step length 4"() -> (w1569:dbl)
                            n137 = local read "dc step length 2"() -> (w1577:dbl)
                            n138 = local read "dc step length 3"() -> (w1572:dbl)
                            n139 = local read "dc step watt 6"() -> (w1560:dbl)
                            n140 = local read "dc step watt 1"() -> (w1582:dbl)
                            n141 = local read "dc step watt 5"() -> (w1565:dbl)
                            n142 = local read "dc step watt 2"() -> (w1576:dbl)
                            n143 = local read "dc step watt 4"() -> (w1568:dbl)
                            n144 = local read "dc step watt 3"() -> (w1573:dbl)
                            n145 = Equal To 0?(x=w1560) -> (x = 0?=w1559:bool)
                            n146 = Equal To 0?(x=w1561) -> (x = 0?=w1558:bool)
                            n147 = Equal To 0?(x=w1565) -> (x = 0?=w1563:bool)
                            n148 = Equal To 0?(x=w1582) -> (x = 0?=w1580:bool)
                            n149 = Equal To 0?(x=w1564) -> (x = 0?=w1562:bool)
                            n150 = Equal To 0?(x=w1576) -> (x = 0?=w1575:bool)
                            n151 = Equal To 0?(x=w1568) -> (x = 0?=w1567:bool)
                            n152 = Equal To 0?(x=w1581) -> (x = 0?=w1579:bool)
                            n153 = Equal To 0?(x=w1573) -> (x = 0?=w1571:bool)
                            n154 = Equal To 0?(x=w1569) -> (x = 0?=w1566:bool)
                            n155 = Equal To 0?(x=w1577) -> (x = 0?=w1574:bool)
                            n156 = Equal To 0?(x=w1572) -> (x = 0?=w1570:bool)
                            n157 = Compound Arithmetic op=OR(w1580, w1579, w1575, w1574, w1571, w1570, w1567, w1566, w1563, w1562, w1559, w1558) -> (w1578:bool)
                          }
                          frame 7 {
                            n158 = local read "dc step length 6"() -> (w1590:dbl)
                            n159 = local read "dc step length 7"() -> (w1585:dbl)
                            n160 = local read "dc step length 5"() -> (w1593:dbl)
                            n161 = local read "dc step length 1"() -> (w1610:dbl)
                            n162 = local read "dc step length 4"() -> (w1598:dbl)
                            n163 = local read "dc step length 2"() -> (w1606:dbl)
                            n164 = local read "dc step length 3"() -> (w1601:dbl)
                            n165 = local read "dc step watt 6"() -> (w1589:dbl)
                            n166 = local read "dc step watt 7"() -> (w1586:dbl)
                            n167 = local read "dc step watt 1"() -> (w1611:dbl)
                            n168 = local read "dc step watt 5"() -> (w1594:dbl)
                            n169 = local read "dc step watt 2"() -> (w1605:dbl)
                            n170 = local read "dc step watt 4"() -> (w1597:dbl)
                            n171 = local read "dc step watt 3"() -> (w1602:dbl)
                            n172 = Equal To 0?(x=w1589) -> (x = 0?=w1588:bool)
                            n173 = Equal To 0?(x=w1586) -> (x = 0?=w1584:bool)
                            n174 = Equal To 0?(x=w1590) -> (x = 0?=w1587:bool)
                            n175 = Equal To 0?(x=w1585) -> (x = 0?=w1583:bool)
                            n176 = Equal To 0?(x=w1594) -> (x = 0?=w1592:bool)
                            n177 = Equal To 0?(x=w1611) -> (x = 0?=w1609:bool)
                            n178 = Equal To 0?(x=w1593) -> (x = 0?=w1591:bool)
                            n179 = Equal To 0?(x=w1605) -> (x = 0?=w1604:bool)
                            n180 = Equal To 0?(x=w1597) -> (x = 0?=w1596:bool)
                            n181 = Equal To 0?(x=w1610) -> (x = 0?=w1608:bool)
                            n182 = Equal To 0?(x=w1602) -> (x = 0?=w1600:bool)
                            n183 = Equal To 0?(x=w1598) -> (x = 0?=w1595:bool)
                            n184 = Equal To 0?(x=w1606) -> (x = 0?=w1603:bool)
                            n185 = Equal To 0?(x=w1601) -> (x = 0?=w1599:bool)
                            n186 = Compound Arithmetic op=OR(w1609, w1608, w1604, w1603, w1600, w1599, w1596, w1595, w1592, w1591, w1588, w1587, w1584, w1583) -> (w1607:bool)
                          }
                          frame 8 {
                            n187 = local read "dc step length 6"() -> (w1623:dbl)
                            n188 = local read "dc step length 7"() -> (w1618:dbl)
                            n189 = local read "dc step length 8"() -> (w1615:dbl)
                            n190 = local read "dc step length 5"() -> (w1626:dbl)
                            n191 = local read "dc step length 1"() -> (w1643:dbl)
                            n192 = local read "dc step length 4"() -> (w1631:dbl)
                            n193 = local read "dc step length 2"() -> (w1639:dbl)
                            n194 = local read "dc step length 3"() -> (w1634:dbl)
                            n195 = local read "dc step watt 6"() -> (w1622:dbl)
                            n196 = local read "dc step watt 7"() -> (w1619:dbl)
                            n197 = local read "dc step watt 8"() -> (w1614:dbl)
                            n198 = local read "dc step watt 1"() -> (w1644:dbl)
                            n199 = local read "dc step watt 5"() -> (w1627:dbl)
                            n200 = local read "dc step watt 2"() -> (w1638:dbl)
                            n201 = local read "dc step watt 4"() -> (w1630:dbl)
                            n202 = local read "dc step watt 3"() -> (w1635:dbl)
                            n203 = Equal To 0?(x=w1622) -> (x = 0?=w1621:bool)
                            n204 = Equal To 0?(x=w1619) -> (x = 0?=w1617:bool)
                            n205 = Equal To 0?(x=w1623) -> (x = 0?=w1620:bool)
                            n206 = Equal To 0?(x=w1618) -> (x = 0?=w1616:bool)
                            n207 = Equal To 0?(x=w1614) -> (x = 0?=w1613:bool)
                            n208 = Equal To 0?(x=w1627) -> (x = 0?=w1625:bool)
                            n209 = Equal To 0?(x=w1615) -> (x = 0?=w1612:bool)
                            n210 = Equal To 0?(x=w1644) -> (x = 0?=w1642:bool)
                            n211 = Equal To 0?(x=w1626) -> (x = 0?=w1624:bool)
                            n212 = Equal To 0?(x=w1638) -> (x = 0?=w1637:bool)
                            n213 = Equal To 0?(x=w1630) -> (x = 0?=w1629:bool)
                            n214 = Equal To 0?(x=w1643) -> (x = 0?=w1641:bool)
                            n215 = Equal To 0?(x=w1635) -> (x = 0?=w1633:bool)
                            n216 = Equal To 0?(x=w1631) -> (x = 0?=w1628:bool)
                            n217 = Equal To 0?(x=w1639) -> (x = 0?=w1636:bool)
                            n218 = Equal To 0?(x=w1634) -> (x = 0?=w1632:bool)
                            n219 = Compound Arithmetic op=OR(w1642, w1641, w1637, w1636, w1633, w1632, w1629, w1628, w1625, w1624, w1621, w1620, w1617, w1616, w1613, w1612) -> (w1640:bool)
                          }
                          frame 9 {
                            n220 = local read "dc step length 1"() -> (w1680:dbl)
                            n221 = local read "dc step length 2"() -> (w1676:dbl)
                            n222 = local read "dc step length 3"() -> (w1671:dbl)
                            n223 = local read "dc step length 4"() -> (w1668:dbl)
                            n224 = local read "dc step length 5"() -> (w1663:dbl)
                            n225 = local read "dc step length 6"() -> (w1660:dbl)
                            n226 = local read "dc step length 7"() -> (w1655:dbl)
                            n227 = local read "dc step length 8"() -> (w1652:dbl)
                            n228 = local read "dc step length 9"() -> (w1647:dbl)
                            n229 = local read "dc step watt 1"() -> (w1681:dbl)
                            n230 = local read "dc step watt 2"() -> (w1675:dbl)
                            n231 = local read "dc step watt 3"() -> (w1672:dbl)
                            n232 = local read "dc step watt 4"() -> (w1667:dbl)
                            n233 = local read "dc step watt 5"() -> (w1664:dbl)
                            n234 = local read "dc step watt 6"() -> (w1659:dbl)
                            n235 = local read "dc step watt 7"() -> (w1656:dbl)
                            n236 = local read "dc step watt 8"() -> (w1651:dbl)
                            n237 = local read "dc step watt 9"() -> (w1648:dbl)
                            n238 = Equal To 0?(x=w1659) -> (x = 0?=w1658:bool)
                            n239 = Equal To 0?(x=w1656) -> (x = 0?=w1654:bool)
                            n240 = Equal To 0?(x=w1660) -> (x = 0?=w1657:bool)
                            n241 = Equal To 0?(x=w1655) -> (x = 0?=w1653:bool)
                            n242 = Equal To 0?(x=w1651) -> (x = 0?=w1650:bool)
                            n243 = Equal To 0?(x=w1664) -> (x = 0?=w1662:bool)
                            n244 = Equal To 0?(x=w1652) -> (x = 0?=w1649:bool)
                            n245 = Equal To 0?(x=w1681) -> (x = 0?=w1679:bool)
                            n246 = Equal To 0?(x=w1663) -> (x = 0?=w1661:bool)
                            n247 = Equal To 0?(x=w1675) -> (x = 0?=w1674:bool)
                            n248 = Equal To 0?(x=w1667) -> (x = 0?=w1666:bool)
                            n249 = Equal To 0?(x=w1648) -> (x = 0?=w1646:bool)
                            n250 = Equal To 0?(x=w1680) -> (x = 0?=w1678:bool)
                            n251 = Equal To 0?(x=w1672) -> (x = 0?=w1670:bool)
                            n252 = Equal To 0?(x=w1668) -> (x = 0?=w1665:bool)
                            n253 = Equal To 0?(x=w1676) -> (x = 0?=w1673:bool)
                            n254 = Equal To 0?(x=w1671) -> (x = 0?=w1669:bool)
                            n255 = Equal To 0?(x=w1647) -> (x = 0?=w1645:bool)
                            n256 = Compound Arithmetic op=OR(w1679, w1678, w1674, w1673, w1670, w1669, w1666, w1665, w1662, w1661, w1658, w1657, w1654, w1653, w1650, w1649, w1646, w1645) -> (w1677:bool)
                          }
                          frame 10 {
                            n257 = local read "dc step length 10"() -> (w1685:dbl)
                            n258 = local read "dc step length 1"() -> (w1721:dbl)
                            n259 = local read "dc step length 2"() -> (w1717:dbl)
                            n260 = local read "dc step length 3"() -> (w1712:dbl)
                            n261 = local read "dc step length 4"() -> (w1709:dbl)
                            n262 = local read "dc step length 5"() -> (w1704:dbl)
                            n263 = local read "dc step length 6"() -> (w1701:dbl)
                            n264 = local read "dc step length 7"() -> (w1696:dbl)
                            n265 = local read "dc step length 8"() -> (w1693:dbl)
                            n266 = local read "dc step length 9"() -> (w1688:dbl)
                            n267 = local read "dc step watt 10"() -> (w1684:dbl)
                            n268 = local read "dc step watt 1"() -> (w1722:dbl)
                            n269 = local read "dc step watt 2"() -> (w1716:dbl)
                            n270 = local read "dc step watt 3"() -> (w1713:dbl)
                            n271 = local read "dc step watt 4"() -> (w1708:dbl)
                            n272 = local read "dc step watt 5"() -> (w1705:dbl)
                            n273 = local read "dc step watt 6"() -> (w1700:dbl)
                            n274 = local read "dc step watt 7"() -> (w1697:dbl)
                            n275 = local read "dc step watt 8"() -> (w1692:dbl)
                            n276 = local read "dc step watt 9"() -> (w1689:dbl)
                            n277 = Equal To 0?(x=w1722) -> (x = 0?=w1720:bool)
                            n278 = Equal To 0?(x=w1721) -> (x = 0?=w1719:bool)
                            n279 = Equal To 0?(x=w1716) -> (x = 0?=w1715:bool)
                            n280 = Equal To 0?(x=w1717) -> (x = 0?=w1714:bool)
                            n281 = Equal To 0?(x=w1713) -> (x = 0?=w1711:bool)
                            n282 = Equal To 0?(x=w1712) -> (x = 0?=w1710:bool)
                            n283 = Equal To 0?(x=w1708) -> (x = 0?=w1707:bool)
                            n284 = Equal To 0?(x=w1709) -> (x = 0?=w1706:bool)
                            n285 = Equal To 0?(x=w1705) -> (x = 0?=w1703:bool)
                            n286 = Equal To 0?(x=w1704) -> (x = 0?=w1702:bool)
                            n287 = Equal To 0?(x=w1700) -> (x = 0?=w1699:bool)
                            n288 = Equal To 0?(x=w1701) -> (x = 0?=w1698:bool)
                            n289 = Equal To 0?(x=w1697) -> (x = 0?=w1695:bool)
                            n290 = Equal To 0?(x=w1696) -> (x = 0?=w1694:bool)
                            n291 = Equal To 0?(x=w1692) -> (x = 0?=w1691:bool)
                            n292 = Equal To 0?(x=w1693) -> (x = 0?=w1690:bool)
                            n293 = Equal To 0?(x=w1689) -> (x = 0?=w1687:bool)
                            n294 = Equal To 0?(x=w1688) -> (x = 0?=w1686:bool)
                            n295 = Equal To 0?(x=w1684) -> (x = 0?=w1683:bool)
                            n296 = Equal To 0?(x=w1685) -> (x = 0?=w1682:bool)
                            n297 = Compound Arithmetic op=OR(w1720, w1719, w1715, w1714, w1711, w1710, w1707, w1706, w1703, w1702, w1699, w1698, w1695, w1694, w1691, w1690, w1687, w1686, w1683, w1682) -> (w1718:bool)
                          }
                        }
                      }
                      frame "rfsputter" {
                        n298 = case shown="10" w1723 {
                          tunnel: [FALSE w1728 w1737 w1750 w1767 w1788 w1813 w1842 w1875 w1912 w1953] -> w1724
                          frame 0, Default {
                          }
                          frame 1 {
                            n299 = local read "rf step length 1"() -> (w1731:dbl)
                            n300 = local read "rf step watt 1"() -> (w1732:dbl)
                            n301 = Equal To 0?(x=w1732) -> (x = 0?=w1730:bool)
                            n302 = Equal To 0?(x=w1731) -> (x = 0?=w1729:bool)
                            n303 = Compound Arithmetic op=OR(w1730, w1729) -> (w1728:bool)
                          }
                          frame 2 {
                            n304 = local read "rf step length 1"() -> (w1740:dbl)
                            n305 = local read "rf step length 2"() -> (w1736:dbl)
                            n306 = local read "rf step watt 1"() -> (w1741:dbl)
                            n307 = local read "rf step watt 2"() -> (w1735:dbl)
                            n308 = Equal To 0?(x=w1741) -> (x = 0?=w1739:bool)
                            n309 = Equal To 0?(x=w1735) -> (x = 0?=w1734:bool)
                            n310 = Equal To 0?(x=w1740) -> (x = 0?=w1738:bool)
                            n311 = Equal To 0?(x=w1736) -> (x = 0?=w1733:bool)
                            n312 = Compound Arithmetic op=OR(w1739, w1738, w1734, w1733) -> (w1737:bool)
                          }
                          frame 3 {
                            n313 = local read "rf step length 1"() -> (w1753:dbl)
                            n314 = local read "rf step length 2"() -> (w1749:dbl)
                            n315 = local read "rf step length 3"() -> (w1744:dbl)
                            n316 = local read "rf step watt 1"() -> (w1754:dbl)
                            n317 = local read "rf step watt 2"() -> (w1748:dbl)
                            n318 = local read "rf step watt 3"() -> (w1745:dbl)
                            n319 = Equal To 0?(x=w1754) -> (x = 0?=w1752:bool)
                            n320 = Equal To 0?(x=w1748) -> (x = 0?=w1747:bool)
                            n321 = Equal To 0?(x=w1753) -> (x = 0?=w1751:bool)
                            n322 = Equal To 0?(x=w1745) -> (x = 0?=w1743:bool)
                            n323 = Equal To 0?(x=w1749) -> (x = 0?=w1746:bool)
                            n324 = Equal To 0?(x=w1744) -> (x = 0?=w1742:bool)
                            n325 = Compound Arithmetic op=OR(w1752, w1751, w1747, w1746, w1743, w1742) -> (w1750:bool)
                          }
                          frame 4 {
                            n326 = local read "rf step length 1"() -> (w1770:dbl)
                            n327 = local read "rf step length 4"() -> (w1758:dbl)
                            n328 = local read "rf step length 2"() -> (w1766:dbl)
                            n329 = local read "rf step length 3"() -> (w1761:dbl)
                            n330 = local read "rf step watt 1"() -> (w1771:dbl)
                            n331 = local read "rf step watt 2"() -> (w1765:dbl)
                            n332 = local read "rf step watt 4"() -> (w1757:dbl)
                            n333 = local read "rf step watt 3"() -> (w1762:dbl)
                            n334 = Equal To 0?(x=w1771) -> (x = 0?=w1769:bool)
                            n335 = Equal To 0?(x=w1765) -> (x = 0?=w1764:bool)
                            n336 = Equal To 0?(x=w1757) -> (x = 0?=w1756:bool)
                            n337 = Equal To 0?(x=w1770) -> (x = 0?=w1768:bool)
                            n338 = Equal To 0?(x=w1762) -> (x = 0?=w1760:bool)
                            n339 = Equal To 0?(x=w1758) -> (x = 0?=w1755:bool)
                            n340 = Equal To 0?(x=w1766) -> (x = 0?=w1763:bool)
                            n341 = Equal To 0?(x=w1761) -> (x = 0?=w1759:bool)
                            n342 = Compound Arithmetic op=OR(w1769, w1768, w1764, w1763, w1760, w1759, w1756, w1755) -> (w1767:bool)
                          }
                          frame 5 {
                            n343 = local read "rf step length 1"() -> (w1791:dbl)
                            n344 = local read "rf step length 2"() -> (w1787:dbl)
                            n345 = local read "rf step length 3"() -> (w1782:dbl)
                            n346 = local read "rf step length 4"() -> (w1779:dbl)
                            n347 = local read "rf step length 5"() -> (w1774:dbl)
                            n348 = local read "rf step watt 1"() -> (w1792:dbl)
                            n349 = local read "rf step watt 2"() -> (w1786:dbl)
                            n350 = local read "rf step watt 3"() -> (w1783:dbl)
                            n351 = local read "rf step watt 4"() -> (w1778:dbl)
                            n352 = local read "rf step watt 5"() -> (w1775:dbl)
                            n353 = Equal To 0?(x=w1792) -> (x = 0?=w1790:bool)
                            n354 = Equal To 0?(x=w1791) -> (x = 0?=w1789:bool)
                            n355 = Equal To 0?(x=w1786) -> (x = 0?=w1785:bool)
                            n356 = Equal To 0?(x=w1787) -> (x = 0?=w1784:bool)
                            n357 = Equal To 0?(x=w1783) -> (x = 0?=w1781:bool)
                            n358 = Equal To 0?(x=w1782) -> (x = 0?=w1780:bool)
                            n359 = Equal To 0?(x=w1778) -> (x = 0?=w1777:bool)
                            n360 = Equal To 0?(x=w1779) -> (x = 0?=w1776:bool)
                            n361 = Equal To 0?(x=w1775) -> (x = 0?=w1773:bool)
                            n362 = Equal To 0?(x=w1774) -> (x = 0?=w1772:bool)
                            n363 = Compound Arithmetic op=OR(w1790, w1789, w1785, w1784, w1781, w1780, w1777, w1776, w1773, w1772) -> (w1788:bool)
                          }
                          frame 6 {
                            n364 = local read "rf step length 3"() -> (w1807:dbl)
                            n365 = local read "rf step length 4"() -> (w1804:dbl)
                            n366 = local read "rf step length 5"() -> (w1799:dbl)
                            n367 = local read "rf step length 6"() -> (w1796:dbl)
                            n368 = local read "rf step length 1"() -> (w1816:dbl)
                            n369 = local read "rf step length 2"() -> (w1812:dbl)
                            n370 = local read "rf step watt 4"() -> (w1803:dbl)
                            n371 = local read "rf step watt 5"() -> (w1800:dbl)
                            n372 = local read "rf step watt 6"() -> (w1795:dbl)
                            n373 = local read "rf step watt 1"() -> (w1817:dbl)
                            n374 = local read "rf step watt 2"() -> (w1811:dbl)
                            n375 = local read "rf step watt 3"() -> (w1808:dbl)
                            n376 = Equal To 0?(x=w1795) -> (x = 0?=w1794:bool)
                            n377 = Equal To 0?(x=w1796) -> (x = 0?=w1793:bool)
                            n378 = Equal To 0?(x=w1800) -> (x = 0?=w1798:bool)
                            n379 = Equal To 0?(x=w1817) -> (x = 0?=w1815:bool)
                            n380 = Equal To 0?(x=w1799) -> (x = 0?=w1797:bool)
                            n381 = Equal To 0?(x=w1811) -> (x = 0?=w1810:bool)
                            n382 = Equal To 0?(x=w1803) -> (x = 0?=w1802:bool)
                            n383 = Equal To 0?(x=w1816) -> (x = 0?=w1814:bool)
                            n384 = Equal To 0?(x=w1808) -> (x = 0?=w1806:bool)
                            n385 = Equal To 0?(x=w1804) -> (x = 0?=w1801:bool)
                            n386 = Equal To 0?(x=w1812) -> (x = 0?=w1809:bool)
                            n387 = Equal To 0?(x=w1807) -> (x = 0?=w1805:bool)
                            n388 = Compound Arithmetic op=OR(w1815, w1814, w1810, w1809, w1806, w1805, w1802, w1801, w1798, w1797, w1794, w1793) -> (w1813:bool)
                          }
                          frame 7 {
                            n389 = local read "rf step length 5"() -> (w1828:dbl)
                            n390 = local read "rf step length 6"() -> (w1825:dbl)
                            n391 = local read "rf step length 7"() -> (w1820:dbl)
                            n392 = local read "rf step length 1"() -> (w1845:dbl)
                            n393 = local read "rf step length 2"() -> (w1841:dbl)
                            n394 = local read "rf step length 3"() -> (w1836:dbl)
                            n395 = local read "rf step length 4"() -> (w1833:dbl)
                            n396 = local read "rf step watt 5"() -> (w1829:dbl)
                            n397 = local read "rf step watt 6"() -> (w1824:dbl)
                            n398 = local read "rf step watt 7"() -> (w1821:dbl)
                            n399 = local read "rf step watt 1"() -> (w1846:dbl)
                            n400 = local read "rf step watt 2"() -> (w1840:dbl)
                            n401 = local read "rf step watt 3"() -> (w1837:dbl)
                            n402 = local read "rf step watt 4"() -> (w1832:dbl)
                            n403 = Equal To 0?(x=w1846) -> (x = 0?=w1844:bool)
                            n404 = Equal To 0?(x=w1845) -> (x = 0?=w1843:bool)
                            n405 = Equal To 0?(x=w1840) -> (x = 0?=w1839:bool)
                            n406 = Equal To 0?(x=w1841) -> (x = 0?=w1838:bool)
                            n407 = Equal To 0?(x=w1837) -> (x = 0?=w1835:bool)
                            n408 = Equal To 0?(x=w1836) -> (x = 0?=w1834:bool)
                            n409 = Equal To 0?(x=w1832) -> (x = 0?=w1831:bool)
                            n410 = Equal To 0?(x=w1833) -> (x = 0?=w1830:bool)
                            n411 = Equal To 0?(x=w1829) -> (x = 0?=w1827:bool)
                            n412 = Equal To 0?(x=w1828) -> (x = 0?=w1826:bool)
                            n413 = Equal To 0?(x=w1824) -> (x = 0?=w1823:bool)
                            n414 = Equal To 0?(x=w1825) -> (x = 0?=w1822:bool)
                            n415 = Equal To 0?(x=w1821) -> (x = 0?=w1819:bool)
                            n416 = Equal To 0?(x=w1820) -> (x = 0?=w1818:bool)
                            n417 = Compound Arithmetic op=OR(w1844, w1843, w1839, w1838, w1835, w1834, w1831, w1830, w1827, w1826, w1823, w1822, w1819, w1818) -> (w1842:bool)
                          }
                          frame 8 {
                            n418 = local read "rf step length 6"() -> (w1858:dbl)
                            n419 = local read "rf step length 7"() -> (w1853:dbl)
                            n420 = local read "rf step length 8"() -> (w1850:dbl)
                            n421 = local read "rf step length 5"() -> (w1861:dbl)
                            n422 = local read "rf step length 1"() -> (w1878:dbl)
                            n423 = local read "rf step length 4"() -> (w1866:dbl)
                            n424 = local read "rf step length 2"() -> (w1874:dbl)
                            n425 = local read "rf step length 3"() -> (w1869:dbl)
                            n426 = local read "rf step watt 6"() -> (w1857:dbl)
                            n427 = local read "rf step watt 7"() -> (w1854:dbl)
                            n428 = local read "rf step watt 8"() -> (w1849:dbl)
                            n429 = local read "rf step watt 5"() -> (w1862:dbl)
                            n430 = local read "rf step watt 1"() -> (w1879:dbl)
                            n431 = local read "rf step watt 2"() -> (w1873:dbl)
                            n432 = local read "rf step watt 4"() -> (w1865:dbl)
                            n433 = local read "rf step watt 3"() -> (w1870:dbl)
                            n434 = Equal To 0?(x=w1857) -> (x = 0?=w1856:bool)
                            n435 = Equal To 0?(x=w1854) -> (x = 0?=w1852:bool)
                            n436 = Equal To 0?(x=w1858) -> (x = 0?=w1855:bool)
                            n437 = Equal To 0?(x=w1853) -> (x = 0?=w1851:bool)
                            n438 = Equal To 0?(x=w1849) -> (x = 0?=w1848:bool)
                            n439 = Equal To 0?(x=w1862) -> (x = 0?=w1860:bool)
                            n440 = Equal To 0?(x=w1850) -> (x = 0?=w1847:bool)
                            n441 = Equal To 0?(x=w1879) -> (x = 0?=w1877:bool)
                            n442 = Equal To 0?(x=w1861) -> (x = 0?=w1859:bool)
                            n443 = Equal To 0?(x=w1873) -> (x = 0?=w1872:bool)
                            n444 = Equal To 0?(x=w1865) -> (x = 0?=w1864:bool)
                            n445 = Equal To 0?(x=w1878) -> (x = 0?=w1876:bool)
                            n446 = Equal To 0?(x=w1870) -> (x = 0?=w1868:bool)
                            n447 = Equal To 0?(x=w1866) -> (x = 0?=w1863:bool)
                            n448 = Equal To 0?(x=w1874) -> (x = 0?=w1871:bool)
                            n449 = Equal To 0?(x=w1869) -> (x = 0?=w1867:bool)
                            n450 = Compound Arithmetic op=OR(w1877, w1876, w1872, w1871, w1868, w1867, w1864, w1863, w1860, w1859, w1856, w1855, w1852, w1851, w1848, w1847) -> (w1875:bool)
                          }
                          frame 9 {
                            n451 = local read "rf step length 1"() -> (w1915:dbl)
                            n452 = local read "rf step length 2"() -> (w1911:dbl)
                            n453 = local read "rf step length 3"() -> (w1906:dbl)
                            n454 = local read "rf step length 4"() -> (w1903:dbl)
                            n455 = local read "rf step length 5"() -> (w1898:dbl)
                            n456 = local read "rf step length 6"() -> (w1895:dbl)
                            n457 = local read "rf step length 7"() -> (w1890:dbl)
                            n458 = local read "rf step length 8"() -> (w1887:dbl)
                            n459 = local read "rf step length 9"() -> (w1882:dbl)
                            n460 = local read "rf step watt 1"() -> (w1916:dbl)
                            n461 = local read "rf step watt 2"() -> (w1910:dbl)
                            n462 = local read "rf step watt 3"() -> (w1907:dbl)
                            n463 = local read "rf step watt 4"() -> (w1902:dbl)
                            n464 = local read "rf step watt 5"() -> (w1899:dbl)
                            n465 = local read "rf step watt 6"() -> (w1894:dbl)
                            n466 = local read "rf step watt 7"() -> (w1891:dbl)
                            n467 = local read "rf step watt 8"() -> (w1886:dbl)
                            n468 = local read "rf step watt 9"() -> (w1883:dbl)
                            n469 = Equal To 0?(x=w1916) -> (x = 0?=w1914:bool)
                            n470 = Equal To 0?(x=w1915) -> (x = 0?=w1913:bool)
                            n471 = Equal To 0?(x=w1910) -> (x = 0?=w1909:bool)
                            n472 = Equal To 0?(x=w1911) -> (x = 0?=w1908:bool)
                            n473 = Equal To 0?(x=w1907) -> (x = 0?=w1905:bool)
                            n474 = Equal To 0?(x=w1906) -> (x = 0?=w1904:bool)
                            n475 = Equal To 0?(x=w1902) -> (x = 0?=w1901:bool)
                            n476 = Equal To 0?(x=w1903) -> (x = 0?=w1900:bool)
                            n477 = Equal To 0?(x=w1899) -> (x = 0?=w1897:bool)
                            n478 = Equal To 0?(x=w1898) -> (x = 0?=w1896:bool)
                            n479 = Equal To 0?(x=w1894) -> (x = 0?=w1893:bool)
                            n480 = Equal To 0?(x=w1895) -> (x = 0?=w1892:bool)
                            n481 = Equal To 0?(x=w1891) -> (x = 0?=w1889:bool)
                            n482 = Equal To 0?(x=w1890) -> (x = 0?=w1888:bool)
                            n483 = Equal To 0?(x=w1886) -> (x = 0?=w1885:bool)
                            n484 = Equal To 0?(x=w1887) -> (x = 0?=w1884:bool)
                            n485 = Equal To 0?(x=w1883) -> (x = 0?=w1881:bool)
                            n486 = Equal To 0?(x=w1882) -> (x = 0?=w1880:bool)
                            n487 = Compound Arithmetic op=OR(w1914, w1913, w1909, w1908, w1905, w1904, w1901, w1900, w1897, w1896, w1893, w1892, w1889, w1888, w1885, w1884, w1881, w1880) -> (w1912:bool)
                          }
                          frame 10 {
                            n488 = local read "rf step length 10"() -> (w1920:dbl)
                            n489 = local read "rf step length 1"() -> (w1956:dbl)
                            n490 = local read "rf step length 2"() -> (w1952:dbl)
                            n491 = local read "rf step length 3"() -> (w1947:dbl)
                            n492 = local read "rf step length 4"() -> (w1944:dbl)
                            n493 = local read "rf step length 5"() -> (w1939:dbl)
                            n494 = local read "rf step length 6"() -> (w1936:dbl)
                            n495 = local read "rf step length 7"() -> (w1931:dbl)
                            n496 = local read "rf step length 8"() -> (w1928:dbl)
                            n497 = local read "rf step length 9"() -> (w1923:dbl)
                            n498 = local read "rf step watt 10"() -> (w1919:dbl)
                            n499 = local read "rf step watt 1"() -> (w1957:dbl)
                            n500 = local read "rf step watt 2"() -> (w1951:dbl)
                            n501 = local read "rf step watt 3"() -> (w1948:dbl)
                            n502 = local read "rf step watt 4"() -> (w1943:dbl)
                            n503 = local read "rf step watt 5"() -> (w1940:dbl)
                            n504 = local read "rf step watt 6"() -> (w1935:dbl)
                            n505 = local read "rf step watt 7"() -> (w1932:dbl)
                            n506 = local read "rf step watt 8"() -> (w1927:dbl)
                            n507 = local read "rf step watt 9"() -> (w1924:dbl)
                            n508 = Equal To 0?(x=w1919) -> (x = 0?=w1918:bool)
                            n509 = Equal To 0?(x=w1920) -> (x = 0?=w1917:bool)
                            n510 = Equal To 0?(x=w1957) -> (x = 0?=w1955:bool)
                            n511 = Equal To 0?(x=w1956) -> (x = 0?=w1954:bool)
                            n512 = Equal To 0?(x=w1951) -> (x = 0?=w1950:bool)
                            n513 = Equal To 0?(x=w1952) -> (x = 0?=w1949:bool)
                            n514 = Equal To 0?(x=w1948) -> (x = 0?=w1946:bool)
                            n515 = Equal To 0?(x=w1947) -> (x = 0?=w1945:bool)
                            n516 = Equal To 0?(x=w1943) -> (x = 0?=w1942:bool)
                            n517 = Equal To 0?(x=w1944) -> (x = 0?=w1941:bool)
                            n518 = Equal To 0?(x=w1940) -> (x = 0?=w1938:bool)
                            n519 = Equal To 0?(x=w1939) -> (x = 0?=w1937:bool)
                            n520 = Equal To 0?(x=w1935) -> (x = 0?=w1934:bool)
                            n521 = Equal To 0?(x=w1936) -> (x = 0?=w1933:bool)
                            n522 = Equal To 0?(x=w1932) -> (x = 0?=w1930:bool)
                            n523 = Equal To 0?(x=w1931) -> (x = 0?=w1929:bool)
                            n524 = Equal To 0?(x=w1927) -> (x = 0?=w1926:bool)
                            n525 = Equal To 0?(x=w1928) -> (x = 0?=w1925:bool)
                            n526 = Equal To 0?(x=w1924) -> (x = 0?=w1922:bool)
                            n527 = Equal To 0?(x=w1923) -> (x = 0?=w1921:bool)
                            n528 = Compound Arithmetic op=OR(w1955, w1954, w1950, w1949, w1946, w1945, w1942, w1941, w1938, w1937, w1934, w1933, w1930, w1929, w1926, w1925, w1922, w1921, w1918, w1917) -> (w1953:bool)
                          }
                        }
                      }
                    }
                  }
                  frame 1 {
                    # "multilayer recipe"
                  }
                }
              }
              frame Enabled {
              }
            }
            n529 = local read "Web Selection"() -> (w1462:u16)
            n530 = local read "Substrate Material"() -> (w1469:string)
            n531 = local read "Recipe Name"() -> (w1470:string)
            n532 = case shown="0, Default" w1462 {
              tunnel: [w1969 w1974] -> w1461
              tunnel: [w1968 w1974] -> w1460
              tunnel: [w1967 w1974] -> w1459
              tunnel: [w1966 w1974] -> w1457
              tunnel: [w1964 w1974] -> w1458
              frame 0, Default {
                n533 = local read "left initial diameter"() -> (w1972:dbl)
                n534 = local read "core diameter"() -> (w1973:dbl)
                n535 = local read "web thickness"() -> (w1971:dbl)
                n536 = local read "tension value"() -> (w1970:dbl)
                n537 = local read "web speed"() -> (w1965:dbl)
                n538 = Equal To 0?(x=w1965) -> (x = 0?=w1964:bool)
                n539 = Equal To 0?(x=w1973) -> (x = 0?=w1969:bool)
                n540 = Equal To 0?(x=w1970) -> (x = 0?=w1966:bool)
                n541 = Equal To 0?(x=w1972) -> (x = 0?=w1968:bool)
                n542 = Equal To 0?(x=w1971) -> (x = 0?=w1967:bool)
              }
              frame 1 {
                w1974 = FALSE
              }
            }
            n543 = Equal?(x=w1470, y=w1468) -> (x = y?=w1464:bool)
            n544 = Equal?(x=w1468, y=w1469) -> (x = y?=w1463:bool)
            n545 = local read "power rf"() -> (w1446:dbl)
            n546 = Equal To 0?(x=w1446) -> ()  [unwired: 1 out]
            n547 = local read "Pressure set mbar"() -> (w1449:dbl)
            n548 = local read "total length error"() -> (w1451:bool)
            n549 = local read "Ar set sccm"() -> (w1450:dbl)
            n550 = Equal To 0?(x=w1450) -> (x = 0?=w1448:bool)
            n551 = Equal To 0?(x=w1449) -> (x = 0?=w1447:bool)
            n552 = Build Array(FALSE, w1464, w1463, w1461, w1460, w1459, w1458, w1457, w1455, w1454, w1453, w1451, w1448, w1447) -> (w1452:bool[])
            n553 = Boolean Array To Number(Boolean array=w1452) -> (number=w1467:u32)
            n554 = Mantissa & Exponent(0:w1467) -> (2:w1466:dbl)  [unwired: 1 out]
            n555 = case shown="13" w1466 {
              tunnel: [TRUE FALSE FALSE FALSE FALSE FALSE FALSE FALSE FALSE FALSE FALSE FALSE FALSE FALSE] -> w1456
              frame 0, Default {
              }
              frame 1 {
                n556 = One Button Dialog(message="Enter Recipe Name !") -> ()  [unwired: 1 in, 1 out]
              }
              frame 2 {
                n557 = One Button Dialog(message="Enter Substrate Material !") -> ()  [unwired: 1 in, 1 out]
              }
              frame 3 {
                n558 = One Button Dialog(message="Enter Core Diameter !") -> ()  [unwired: 1 in, 1 out]
              }
              frame 4 {
                n559 = One Button Dialog(message="Enter Left Initial Diameter !") -> ()  [unwired: 1 in, 1 out]
              }
              frame 5 {
                n560 = One Button Dialog(message="Enter Web Thickness !") -> ()  [unwired: 1 in, 1 out]
              }
              frame 6 {
                n561 = One Button Dialog(message="Enter Web Speed !") -> ()  [unwired: 1 in, 1 out]
              }
              frame 7 {
                n562 = One Button Dialog(message="Enter Tension Value !") -> ()  [unwired: 1 in, 1 out]
              }
              frame 8 {
                n563 = One Button Dialog(message="Enter Microwave Power !") -> ()  [unwired: 1 in, 1 out]
              }
              frame 9 {
                n564 = One Button Dialog(message="Check DC Step Length(s) and Power(s) !") -> ()  [unwired: 1 in, 1 out]
              }
              frame 10 {
                n565 = One Button Dialog(message="Enter RF Power !") -> ()  [unwired: 1 in, 1 out]
              }
              frame 11 {
                n566 = One Button Dialog(message="Check Step Length(s) !") -> ()  [unwired: 1 in, 1 out]
              }
              frame 12 {
                n567 = One Button Dialog(message="Enter Argon Flow !") -> ()  [unwired: 1 in, 1 out]
              }
              frame 13 {
                n568 = One Button Dialog(message="Enter Pressure  !") -> ()  [unwired: 1 in, 1 out]
              }
            }
            "done" <- w1456
          }
        }
        n569 = case shown="True" "CALCULATE" {
          frame False {
          }
          frame True {
            n570 = stacked-sequence {
              frame #0 {
                n571 = local write "total length"(0.0 ("total length")) -> ()
                "left diameter after roll" <- "left initial diameter"
              }
              frame #1 {
                n572 = while {
                  i -> [w1436]
                  stop <- w1435 stop-if-true
                  n573 = local read "left diameter after roll"() -> (w1434:dbl)
                  n574 = local read "web thickness"() -> (w1432:dbl)
                  n575 = Wait Until Next ms Multiple(millisecond multiple=u32 100) -> ()  [unwired: 1 out]
                  n576 = local read "core diameter"() -> (w1431:dbl)
                  n577 = Multiply(x=w1432, y=0.002) -> (x*y=w1442:dbl)
                  n578 = Multiply(x=3.141592653589793, y=w1434) -> (x*y=w1425:dbl)
                  n579 = Subtract(x=w1434, y=w1442) -> (x-y=w1441:dbl)
                  n580 = local read "CALCULATE"() -> (w1428:bool)
                  n581 = local write "left diameter after roll"(w1441) -> ()
                  n582 = Divide(x=w1425, y=10.0) -> (x/y=w1427:dbl)
                  n583 = Less Or Equal?(x=w1441, y=w1431) -> (x <= y?=w1437:bool)
                  n584 = local read "total length"() -> (w1439:dbl)
                  n585 = Not(x=w1428) -> (.not. x?=w1429:bool)
                  n586 = Greater Or Equal?(x=w1436, y=600) -> (x >= y?=w1433:bool)
                  n587 = Add(x=w1427, y=w1439) -> (x+y=w1440:dbl)
                  n588 = local write "total length"(w1440) -> ()
                  n589 = Compound Arithmetic op=OR(w1437, w1433, w1429) -> (w1435:bool)
                }
              }
              frame #2 {
                n590 = local write "CALCULATE"(FALSE ("CALCULATE")) -> ()
              }
            }
          }
        }
        n591 = local read "web speed"() -> (w1342:dbl)
        n592 = local read "single process selection"() -> (w1352:enum32{"microwave", "dcsputter", "rfsputter"})
        n593 = local read "Recipe Selection"() -> (w1364:u16)
        n594 = local read "Web Selection"() -> (w1360:u16)
        n595 = Equal?(x=w1364, y=u16 1) -> (x = y?=w1362:bool)
        n596 = Equal?(x=w1360, y=u16 1) -> (x = y?=w1359:bool)
        n597 = In Range and Coerce(upper limit=550.0 ("y"), x=w1342, lower limit=0.0 ("y")) -> (coerced(x)=w1339:dbl)  [unwired: 1 out]
        n598 = case shown="\"rfsputter\"" w1352 {
          tunnel: [T3."Microwave                " ("single process selection") T3."DC Sputter                   " ("single process selection") T3."RF Sputter                         " ("single process selection")] -> w1351
          tunnel: [FALSE TRUE FALSE] -> w1349
          tunnel: [FALSE FALSE TRUE] -> w1348
          frame "microwave", Default {
          }
          frame "dcsputter" {
          }
          frame "rfsputter" {
          }
        }
        n599 = case shown="True" w1362 {
          tunnel: [T2."Single Recipe                                    " ("recipe selection") T2."Multilayer Recipe                                      " ("recipe selection")] -> w1358
          frame False {
          }
          frame True {
          }
        }
        n600 = case shown="False" w1359 {
          tunnel: [T1."Web                                                    " ("web-other tab") T1."Other                                                      " ("web-other tab")] -> w1357
          frame False {
          }
          frame True {
          }
        }
        n601 = local write "web speed"(w1339) -> ()
        n602 = property on="recipe selection" class="TabCtl (strict)"("Value"=w1358) -> ()  [unwired: 2 in, 2 out]
        n603 = property on="web-other tab" class="TabCtl (strict)"("Value"=w1357) -> ()  [unwired: 2 in, 2 out]
        n604 = property on="single process selection" class="TabCtl (strict)"("Value"=w1351) -> ()  [unwired: 2 in, 2 out]
        n605 = property on="steplist tab DC" class="TabCtl (strict)"("Visible"=w1349) -> ()  [unwired: 2 in, 2 out]
        n606 = property on="steplist tab RF" class="TabCtl (strict)"("Visible"=w1348) -> ()  [unwired: 2 in, 2 out]
        n607 = local read "single process selection"() -> (w1347:enum32{"microwave", "dcsputter", "rfsputter"})
        n608 = case shown="\"dcsputter\"" w1347 {
          tunnel: [0.0 w1382 w1406] -> w1356
          frame "microwave", Default {
          }
          frame "rfsputter" {
            n609 = Compound Arithmetic op=ADD("rf step length 1", "rf step length 2", "rf step length 3", "rf step length 4", "rf step length 5", "rf step length 6", "rf step length 7", "rf step length 8", "rf step length 9", "rf step length 10", "rf step length 11", "rf step length 12", "rf step length 13", "rf step length 14", "rf step length 15", "rf step length 16", "rf step length 17", "rf step length 18", "rf step length 19", "rf step length 20") -> (w1382:dbl)
          }
          frame "dcsputter" {
            n610 = Compound Arithmetic op=ADD("dc step length 1", "dc step length 2", "dc step length 3", "dc step length 4", "dc step length 5", "dc step length 6", "dc step length 7", "dc step length 8", "dc step length 9", "dc step length 10", "dc step length 11", "dc step length 12", "dc step length 13", "dc step length 14", "dc step length 15", "dc step length 16", "dc step length 17", "dc step length 18", "dc step length 19", "dc step length 20") -> (w1406:dbl)
          }
        }
        n611 = case shown="True" "CANCEL" {
          tunnel: [FALSE w1367] -> w1344
          frame False {
          }
          frame True {
            n612 = stacked-sequence {
              tunnel: [_ TRUE] -> w1367
              frame #0 {
                n613 = Wait (ms)(milliseconds to wait=u32 500) -> ()  [unwired: 1 out]
              }
              frame #1 {
                w1370 = FALSE ("CALCULATE")
                n614 = local write "CANCEL"(w1370) -> ()
                n615 = local write "CALCULATE"(w1370) -> ()
              }
            }
          }
        }
        n616 = local read "total length"() -> (w1353:dbl)
        n617 = local read "done"() -> (w1346:bool)
        n618 = Greater?(x=w1356, y=w1353) -> ()  [unwired: 1 out]
        n619 = Compound Arithmetic op=OR(w1346, w1344) -> (w1354:bool)
        "total length error" <- FALSE ("total length error")
      }
      n620 = while {
        stop <- w466 stop-if-true
        n621 = local read "done"() -> (w463:bool)
        n622 = Wait Until Next ms Multiple(millisecond multiple=u32 300) -> ()  [unwired: 1 out]
        n623 = case shown="True" w463 {
          tunnel: [FALSE w471] -> w465
          frame False {
          }
          frame True {
            n624 = stacked-sequence {
              seq-local: [w500 _ _ _ _ _ _ _] -> [_ w576 _ _ _ _ _ _]
              seq-local: [_ w574 _ _ _ _ _ _] -> [_ _ w770 _ _ _ _ _]
              seq-local: [_ _ w769 _ _ _ _ _] -> [_ _ _ w882 _ _ _ _]
              seq-local: [_ _ _ w881 _ _ _ _] -> [_ _ _ _ w1036 _ _ _]
              seq-local: [_ _ _ _ w1035 _ _ _] -> [_ _ _ _ _ w1257 _ _]
              seq-local: [_ _ _ _ _ w1256 _ _] -> [_ _ _ _ _ _ w1322 _]
              tunnel: [_ _ _ _ _ _ _ TRUE] -> w471
              frame #0 {
                w478 = "\t"
                w485 = "\t"
                w492 = "\t"
                w496 = "\t"
                w503 = "\r\n"
                w511 = "\r\n"
                w512 = "\t"
                n625 = local read "Recipe Selection"() -> (w509:u16)
                n626 = local read "Web Selection"() -> (w506:u16)
                n627 = Equal?(x=w509, y=u16 0) -> (x = y?=w508:bool)
                n628 = Equal?(x=w506, y=u16 0) -> (x = y?=w507:bool)
                n629 = local read "core diameter"() -> (w501:dbl)
                n630 = case shown="False" w508 {
                  tunnel: ["Multilayer Recipe" ("string") "Single Recipe" ("string")] -> w482
                  frame False {
                  }
                  frame True {
                  }
                }
                n631 = case shown="False" w507 {
                  tunnel: ["Other" ("string") "Web" ("string")] -> w476
                  frame False {
                  }
                  frame True {
                  }
                }
                n632 = local read "Substrate Material"() -> (w493:string)
                n633 = Number To Decimal String(number=w501) -> (decimal integer string=w472:string)  [unwired: 1 in]
                n634 = local read "Recipe Name"() -> (w514:string)
                n635 = Concatenate Strings(w503, w503) -> (w502:string)
                n636 = Concatenate Strings("Core Diameter(mm)" ("string"), w492, w492, w492, ":" ("string"), "\t", w472, "\r\n") -> (w474:string)
                n637 = Concatenate Strings(w511, w511) -> (w504:string)
                n638 = Concatenate Strings("Recipe Selection" ("string"), w485, w485, w485, ":" ("string"), "\t", w482, "\r\n") -> (w484:string)
                n639 = Concatenate Strings("Recipe Name" ("string"), w512, w512, w512, ":" ("string"), "\t", w514, "\r\n") -> (w515:string)
                n640 = Concatenate Strings("Substrate Material" ("string"), w496, w496, w496, ":" ("string"), "\t", w493, "\r\n") -> (w494:string)
                n641 = Concatenate Strings("Web Selection" ("string"), w478, w478, w478, ":" ("string"), "\t", w476, "\r\n") -> (w475:string)
                n642 = Concatenate Strings(w515, w494, w504, w484, w475, w502, w474) -> (w500:string)
              }
              frame #1 {
                w532 = "\t"
                w539 = "\t"
                w546 = "\t"
                w553 = "\t"
                w560 = "\t"
                w566 = "\t"
                w568 = "\r\n"
                w578 = "\r\n"
                w580 = "\r\n"
                n643 = local read "single process selection"() -> (w570:enum32{"microwave", "dcsputter", "rfsputter"})
                n644 = local read "web thickness"() -> (w573:dbl)
                n645 = local read "left initial diameter"() -> (w524:dbl)
                n646 = case shown="\"dcsputter\"" w570 {
                  tunnel: ["Microwave" ("string") "DC Sputter" ("string") "RF Sputter" ("string")] -> w533
                  tunnel: [FALSE TRUE FALSE] -> w569
                  frame "microwave", Default {
                  }
                  frame "dcsputter" {
                  }
                  frame "rfsputter" {
                  }
                }
                n647 = local read "web speed"() -> (w572:dbl)
                n648 = local read "tension value"() -> (w571:dbl)
                n649 = Number To Decimal String(number=w573) -> (decimal integer string=w556:string)  [unwired: 1 in]
                n650 = Format Into String(format string="%.;%f", w524) -> (resulting string=w523:string)  [unwired: 2 in, 1 out]
                n651 = Number To Decimal String(number=w572) -> (decimal integer string=w547:string)  [unwired: 1 in]
                n652 = Number To Decimal String(number=w571) -> (decimal integer string=w540:string)  [unwired: 1 in]
                n653 = Concatenate Strings(w578, w578) -> (w577:string)
                n654 = Concatenate Strings("Web Thickness(µm)" ("string"), w560, w560, w560, ":" ("string"), "\t", w556, "\r\n") -> (w555:string)
                n655 = case shown="True" w569 {
                  tunnel: ["NULL" ("string") w582] -> w526
                  frame False {
                  }
                  frame True {
                    n656 = local read "DC Sputter Chamber Selection"() -> (w583:enum32{"chamber II", "chamber III"})
                    n657 = case shown="\"chamber II\", Default" w583 {
                      tunnel: ["II" ("string") "III" ("string")] -> w582
                      frame "chamber II", Default {
                      }
                      frame "chamber III" {
                      }
                    }
                  }
                }
                n658 = Concatenate Strings(w580, w580) -> (w579:string)
                n659 = Concatenate Strings("Web Speed(cm/min)" ("string"), w553, w553, w553, ":" ("string"), "\t", w547, "\r\n") -> (w549:string)
                n660 = Concatenate Strings("Tension Value(N)" ("string"), w546, w546, w546, ":" ("string"), "\t", w540, "\r\n") -> (w542:string)
                n661 = Concatenate Strings("Left Initial Diameter(mm)" ("string"), w566, w566, w566, ":" ("string"), "\t", w523, "\r\n") -> (w562:string)
                n662 = Concatenate Strings("Single Process Selection" ("string"), w539, w539, w539, ":" ("string"), "\t", w533, "\r\n") -> (w535:string)
                n663 = Concatenate Strings(w568, w568) -> (w567:string)
                n664 = Concatenate Strings("Chamber Selection" ("string"), w532, w532, w532, ":" ("string"), "\t", w526, "\r\n") -> (w528:string)
                n665 = Concatenate Strings(w562, w555, w579, w549, w542, w577, w535, w528, w567) -> (w575:string)
                n666 = Concatenate Strings(w576, w575) -> (w574:string)
              }
              frame #2 {
                w643 = "\t"
                w638 = "\t"
                w633 = "\t"
                w628 = "\t"
                w623 = "\t"
                w618 = "\t"
                w613 = "\t"
                w608 = "\t"
                w603 = "\t"
                w598 = "\t"
                w683 = "\t"
                w675 = "\t"
                w728 = "\t"
                w742 = "\t"
                w747 = "\t"
                w739 = "\t"
                w734 = "\t"
                w755 = "\t"
                w750 = "\t"
                w758 = "\t"
                w763 = "\t"
                w766 = "\r\n"
                w768 = "\r\n"
                w774 = "\r\n"
                n667 = local read "dc step watt 4"() -> (w753:dbl)
                n668 = local read "dc step watt 1"() -> (w761:dbl)
                n669 = local read "dc step watt 2"() -> (w760:dbl)
                n670 = local read "dc step watt 3"() -> (w752:dbl)
                n671 = local read "dc step watt 5"() -> (w730:dbl)
                n672 = local read "dc step watt 14"() -> (w672:dbl)
                n673 = local read "dc step watt 12"() -> (w673:dbl)
                n674 = local read "dc step watt 13"() -> (w671:dbl)
                n675 = local read "dc step watt 11"() -> (w674:dbl)
                n676 = local read "dc step watt 15"() -> (w665:dbl)
                n677 = Number To Decimal String(number=w753) -> (decimal integer string=w697:string)  [unwired: 1 in]
                n678 = Number To Decimal String(number=w760) -> (decimal integer string=w701:string)  [unwired: 1 in]
                n679 = Number To Decimal String(number=w752) -> (decimal integer string=w699:string)  [unwired: 1 in]
                n680 = Number To Decimal String(number=w761) -> (decimal integer string=w703:string)  [unwired: 1 in]
                n681 = Number To Decimal String(number=w730) -> (decimal integer string=w695:string)  [unwired: 1 in]
                n682 = Number To Decimal String(number=w672) -> (decimal integer string=w651:string)  [unwired: 1 in]
                n683 = Number To Decimal String(number=w673) -> (decimal integer string=w653:string)  [unwired: 1 in]
                n684 = Number To Decimal String(number=w671) -> (decimal integer string=w652:string)  [unwired: 1 in]
                n685 = Number To Decimal String(number=w674) -> (decimal integer string=w654:string)  [unwired: 1 in]
                n686 = Number To Decimal String(number=w665) -> (decimal integer string=w650:string)  [unwired: 1 in]
                n687 = local read "power microwave"() -> (w772:dbl)
                n688 = Number To Decimal String(number=w772) -> (decimal integer string=w678:string)  [unwired: 1 in]
                n689 = Concatenate Strings("DC Step 4 power" ("string"), w755, w755, w755, ":" ("string"), "\t", w697, "\r\n") -> (w723:string)
                n690 = Concatenate Strings("DC Step 5 power" ("string"), w728, w728, w728, ":" ("string"), "\t", w695, "\r\n") -> (w722:string)
                n691 = Concatenate Strings("DC Step 2 power" ("string"), w758, w758, w758, ":" ("string"), "\t", w701, "\r\n") -> (w725:string)
                n692 = Concatenate Strings("DC Step 3 power" ("string"), w750, w750, w750, ":" ("string"), "\t", w699, "\r\n") -> (w724:string)
                n693 = Concatenate Strings("DC Step 1 power" ("string"), w763, w763, w763, ":" ("string"), "\t", w703, "\r\n") -> (w726:string)
                n694 = Concatenate Strings("DC Step 14 power" ("string"), w613, w613, w613, ":" ("string"), "\t", w651, "\r\n") -> (w661:string)
                n695 = Concatenate Strings("DC Step 15 power" ("string"), w638, w638, w638, ":" ("string"), "\t", w650, "\r\n") -> (w660:string)
                n696 = Concatenate Strings("DC Step 12 power" ("string"), w603, w603, w603, ":" ("string"), "\t", w653, "\r\n") -> (w663:string)
                n697 = Concatenate Strings("DC Step 13 power" ("string"), w608, w608, w608, ":" ("string"), "\t", w652, "\r\n") -> (w662:string)
                n698 = Concatenate Strings("DC Step 11 power" ("string"), w598, w598, w598, ":" ("string"), "\t", w654, "\r\n") -> (w664:string)
                n699 = Concatenate Strings("DC Power Steps(power-length)" ("string"), w766, w766) -> (w765:string)
                n700 = Concatenate Strings(w726, w725, w724, w723, w722) -> (w715:string)
                n701 = Concatenate Strings(w774, w774) -> (w773:string)
                n702 = Concatenate Strings(w664, w663, w662, w661, w660) -> (w593:string)
                n703 = Concatenate Strings(w768, w768) -> (w684:string)
                n704 = Concatenate Strings("Microwave Power(watt)" ("string"), w683, w683, w683, ":" ("string"), "\t", w678, "\r\n") -> (w679:string)
                n705 = local read "dc step watt 10"() -> (w731:dbl)
                n706 = local read "dc step watt 9"() -> (w744:dbl)
                n707 = local read "dc step watt 7"() -> (w737:dbl)
                n708 = local read "dc step watt 8"() -> (w745:dbl)
                n709 = local read "dc step watt 6"() -> (w736:dbl)
                n710 = local read "dc step watt 19"() -> (w669:dbl)
                n711 = local read "dc step watt 20"() -> (w666:dbl)
                n712 = local read "dc step watt 17"() -> (w668:dbl)
                n713 = local read "dc step watt 18"() -> (w670:dbl)
                n714 = local read "dc step watt 16"() -> (w667:dbl)
                n715 = Number To Decimal String(number=w744) -> (decimal integer string=w691:string)  [unwired: 1 in]
                n716 = Number To Decimal String(number=w731) -> (decimal integer string=w693:string)  [unwired: 1 in]
                n717 = Number To Decimal String(number=w737) -> (decimal integer string=w687:string)  [unwired: 1 in]
                n718 = Number To Decimal String(number=w745) -> (decimal integer string=w689:string)  [unwired: 1 in]
                n719 = Number To Decimal String(number=w736) -> (decimal integer string=w685:string)  [unwired: 1 in]
                n720 = Number To Decimal String(number=w669) -> (decimal integer string=w648:string)  [unwired: 1 in]
                n721 = Number To Decimal String(number=w666) -> (decimal integer string=w649:string)  [unwired: 1 in]
                n722 = Number To Decimal String(number=w668) -> (decimal integer string=w646:string)  [unwired: 1 in]
                n723 = Number To Decimal String(number=w670) -> (decimal integer string=w647:string)  [unwired: 1 in]
                n724 = Number To Decimal String(number=w667) -> (decimal integer string=w645:string)  [unwired: 1 in]
                n725 = Concatenate Strings("DC Step 9 power" ("string"), w742, w742, w742, ":" ("string"), "\t", w691, "\r\n") -> (w718:string)
                n726 = Concatenate Strings("DC Step 10 power" ("string"), w675, w675, w675, ":" ("string"), "\t", w693, "\r\n") -> (w717:string)
                n727 = Concatenate Strings("DC Step 7 power" ("string"), w739, w739, w739, ":" ("string"), "\t", w687, "\r\n") -> (w720:string)
                n728 = Concatenate Strings("DC Step 8 power" ("string"), w747, w747, w747, ":" ("string"), "\t", w689, "\r\n") -> (w719:string)
                n729 = Concatenate Strings("DC Step 6 power" ("string"), w734, w734, w734, ":" ("string"), "\t", w685, "\r\n") -> (w721:string)
                n730 = Concatenate Strings("DC Step 19 power" ("string"), w633, w633, w633, ":" ("string"), "\t", w648, "\r\n") -> (w656:string)
                n731 = Concatenate Strings("DC Step 20 power" ("string"), w643, w643, w643, ":" ("string"), "\t", w649, "\r\n") -> (w655:string)
                n732 = Concatenate Strings("DC Step 17 power" ("string"), w623, w623, w623, ":" ("string"), "\t", w646, "\r\n") -> (w658:string)
                n733 = Concatenate Strings("DC Step 18 power" ("string"), w628, w628, w628, ":" ("string"), "\t", w647, "\r\n") -> (w657:string)
                n734 = Concatenate Strings("DC Step 16 power" ("string"), w618, w618, w618, ":" ("string"), "\t", w645, "\r\n") -> (w659:string)
                n735 = Concatenate Strings(w659, w658, w657, w656, w655) -> (w594:string)
                n736 = Concatenate Strings(w593, w594) -> (w592:string)
                n737 = Concatenate Strings(w721, w720, w719, w718, w717, w592) -> (w716:string)
                n738 = Concatenate Strings(w679, w684, w773, w765, w715, w716) -> (w771:string)
                n739 = Concatenate Strings(w770, w771) -> (w769:string)
              }
              frame #3 {
                w817 = "\t"
                w814 = "\t"
                w812 = "\t"
                w810 = "\t"
                w779 = "\t"
                w856 = "\t"
                w854 = "\t"
                w852 = "\t"
                w849 = "\t"
                w850 = "\t"
                w879 = "\r\n"
                w859 = "\t"
                w870 = "\t"
                w862 = "\t"
                w864 = "\t"
                w866 = "\t"
                w867 = "\t"
                w872 = "\t"
                w874 = "\t"
                w877 = "\t"
                w876 = "\t"
                n740 = local read "dc step length 4"() -> (w937:dbl)
                n741 = local read "dc step length 2"() -> (w940:dbl)
                n742 = local read "dc step length 3"() -> (w936:dbl)
                n743 = local read "dc step length 1"() -> (w941:dbl)
                n744 = local read "dc step length 5"() -> (w924:dbl)
                n745 = local read "dc step length 14"() -> (w823:dbl)
                n746 = local read "dc step length 12"() -> (w820:dbl)
                n747 = local read "dc step length 13"() -> (w824:dbl)
                n748 = local read "dc step length 11"() -> (w819:dbl)
                n749 = local read "dc step length 15"() -> (w826:dbl)
                n750 = Number To Decimal String(number=w937) -> (decimal integer string=w895:string)  [unwired: 1 in]
                n751 = Number To Decimal String(number=w940) -> (decimal integer string=w899:string)  [unwired: 1 in]
                n752 = Number To Decimal String(number=w936) -> (decimal integer string=w897:string)  [unwired: 1 in]
                n753 = Number To Decimal String(number=w941) -> (decimal integer string=w901:string)  [unwired: 1 in]
                n754 = Number To Decimal String(number=w924) -> (decimal integer string=w893:string)  [unwired: 1 in]
                n755 = Number To Decimal String(number=w823) -> (decimal integer string=w845:string)  [unwired: 1 in]
                n756 = Number To Decimal String(number=w820) -> (decimal integer string=w841:string)  [unwired: 1 in]
                n757 = Number To Decimal String(number=w824) -> (decimal integer string=w843:string)  [unwired: 1 in]
                n758 = Number To Decimal String(number=w819) -> (decimal integer string=w839:string)  [unwired: 1 in]
                n759 = Number To Decimal String(number=w826) -> (decimal integer string=w847:string)  [unwired: 1 in]
                n760 = Concatenate Strings("DC Step 4 length" ("string"), w872, w872, w872, ":" ("string"), "\t", w895, "\r\n") -> (w919:string)
                n761 = Concatenate Strings("DC Step 5 length" ("string"), w870, w870, w870, ":" ("string"), "\t", w893, "\r\n") -> (w918:string)
                n762 = Concatenate Strings("DC Step 2 length" ("string"), w877, w877, w877, ":" ("string"), "\t", w899, "\r\n") -> (w921:string)
                n763 = Concatenate Strings("DC Step 3 length" ("string"), w874, w874, w874, ":" ("string"), "\t", w897, "\r\n") -> (w920:string)
                n764 = Concatenate Strings("DC Step 1 length" ("string"), w876, w876, w876, ":" ("string"), "\t", w901, "\r\n") -> (w922:string)
                n765 = Concatenate Strings("DC Step 14 length" ("string"), w854, w854, w854, ":" ("string"), "\t", w845, "\r\n") -> (w831:string)
                n766 = Concatenate Strings("DC Step 15 length" ("string"), w856, w856, w856, ":" ("string"), "\t", w847, "\r\n") -> (w832:string)
                n767 = Concatenate Strings("DC Step 12 length" ("string"), w849, w849, w849, ":" ("string"), "\t", w841, "\r\n") -> (w829:string)
                n768 = Concatenate Strings("DC Step 13 length" ("string"), w852, w852, w852, ":" ("string"), "\t", w843, "\r\n") -> (w830:string)
                n769 = Concatenate Strings("DC Step 11 length" ("string"), w850, w850, w850, ":" ("string"), "\t", w839, "\r\n") -> (w828:string)
                n770 = Concatenate Strings(w922, w921, w920, w919, w918) -> (w880:string)
                n771 = Concatenate Strings(w828, w829, w830, w831, w832) -> (w777:string)
                n772 = local read "dc step length 10"() -> (w925:dbl)
                n773 = local read "dc step length 9"() -> (w932:dbl)
                n774 = local read "dc step length 7"() -> (w929:dbl)
                n775 = local read "dc step length 8"() -> (w933:dbl)
                n776 = local read "dc step length 6"() -> (w928:dbl)
                n777 = local read "dc step length 19"() -> (w782:dbl)
                n778 = local read "dc step length 20"() -> (w789:dbl)
                n779 = local read "dc step length 17"() -> (w785:dbl)
                n780 = local read "dc step length 18"() -> (w781:dbl)
                n781 = local read "dc step length 16"() -> (w786:dbl)
                n782 = Number To Decimal String(number=w932) -> (decimal integer string=w889:string)  [unwired: 1 in]
                n783 = Number To Decimal String(number=w925) -> (decimal integer string=w891:string)  [unwired: 1 in]
                n784 = Number To Decimal String(number=w929) -> (decimal integer string=w885:string)  [unwired: 1 in]
                n785 = Number To Decimal String(number=w933) -> (decimal integer string=w887:string)  [unwired: 1 in]
                n786 = Number To Decimal String(number=w928) -> (decimal integer string=w883:string)  [unwired: 1 in]
                n787 = Number To Decimal String(number=w782) -> (decimal integer string=w803:string)  [unwired: 1 in]
                n788 = Number To Decimal String(number=w789) -> (decimal integer string=w801:string)  [unwired: 1 in]
                n789 = Number To Decimal String(number=w785) -> (decimal integer string=w807:string)  [unwired: 1 in]
                n790 = Number To Decimal String(number=w781) -> (decimal integer string=w805:string)  [unwired: 1 in]
                n791 = Number To Decimal String(number=w786) -> (decimal integer string=w809:string)  [unwired: 1 in]
                n792 = Concatenate Strings("DC Step 9 length" ("string"), w862, w862, w862, ":" ("string"), "\t", w889, "\r\n") -> (w914:string)
                n793 = Concatenate Strings("DC Step 10 length" ("string"), w859, w859, w859, ":" ("string"), "\t", w891, "\r\n") -> (w913:string)
                n794 = Concatenate Strings("DC Step 7 length" ("string"), w866, w866, w866, ":" ("string"), "\t", w885, "\r\n") -> (w916:string)
                n795 = Concatenate Strings("DC Step 8 length" ("string"), w864, w864, w864, ":" ("string"), "\t", w887, "\r\n") -> (w915:string)
                n796 = Concatenate Strings("DC Step 6 length" ("string"), w867, w867, w867, ":" ("string"), "\t", w883, "\r\n") -> (w917:string)
                n797 = Concatenate Strings("DC Step 19 length" ("string"), w814, w814, w814, ":" ("string"), "\t", w803, "\r\n") -> (w793:string)
                n798 = Concatenate Strings("DC Step 20 length" ("string"), w817, w817, w817, ":" ("string"), "\t", w801, "\r\n") -> (w794:string)
                n799 = Concatenate Strings("DC Step 17 length" ("string"), w810, w810, w810, ":" ("string"), "\t", w807, "\r\n") -> (w791:string)
                n800 = Concatenate Strings("DC Step 18 length" ("string"), w812, w812, w812, ":" ("string"), "\t", w805, "\r\n") -> (w792:string)
                n801 = Concatenate Strings("DC Step 16 length" ("string"), w779, w779, w779, ":" ("string"), "\t", w809, "\r\n") -> (w790:string)
                n802 = Concatenate Strings(w917, w916, w915, w914, w913) -> (w858:string)
                n803 = Concatenate Strings(w790, w791, w792, w793, w794) -> (w776:string)
                n804 = Concatenate Strings(w777, w776) -> (w775:string)
                n805 = Concatenate Strings(w879, w879, w880, w858, w775) -> (w943:string)
                n806 = Concatenate Strings(w882, w943) -> (w881:string)
              }
              frame #4 {
                w1024 = "\t"
                w980 = "\t"
                w985 = "\t"
                w990 = "\t"
                w995 = "\t"
                w1000 = "\t"
                w1005 = "\t"
                w1010 = "\t"
                w1015 = "\t"
                w1020 = "\t"
                w1031 = "\r\n"
                w1033 = "\r\n"
                w1027 = "\t"
                w1080 = "\t"
                w1075 = "\t"
                w1070 = "\t"
                w1065 = "\t"
                w1060 = "\t"
                w1055 = "\t"
                w1050 = "\t"
                w1045 = "\t"
                w1040 = "\t"
                n807 = local read "rf step watt 10"() -> (w1106:dbl)
                n808 = local read "rf step watt 9"() -> (w1109:dbl)
                n809 = local read "rf step watt 7"() -> (w1108:dbl)
                n810 = local read "rf step watt 8"() -> (w1110:dbl)
                n811 = local read "rf step watt 6"() -> (w1107:dbl)
                n812 = local read "rf step watt 4"() -> (w1112:dbl)
                n813 = local read "rf step watt 2"() -> (w1113:dbl)
                n814 = local read "rf step watt 3"() -> (w1111:dbl)
                n815 = local read "rf step watt 1"() -> (w1114:dbl)
                n816 = local read "rf step watt 5"() -> (w1105:dbl)
                n817 = Number To Decimal String(number=w1109) -> (decimal integer string=w1088:string)  [unwired: 1 in]
                n818 = Number To Decimal String(number=w1106) -> (decimal integer string=w1089:string)  [unwired: 1 in]
                n819 = Number To Decimal String(number=w1108) -> (decimal integer string=w1086:string)  [unwired: 1 in]
                n820 = Number To Decimal String(number=w1110) -> (decimal integer string=w1087:string)  [unwired: 1 in]
                n821 = Number To Decimal String(number=w1107) -> (decimal integer string=w1085:string)  [unwired: 1 in]
                n822 = Number To Decimal String(number=w1112) -> (decimal integer string=w1091:string)  [unwired: 1 in]
                n823 = Number To Decimal String(number=w1113) -> (decimal integer string=w1093:string)  [unwired: 1 in]
                n824 = Number To Decimal String(number=w1111) -> (decimal integer string=w1092:string)  [unwired: 1 in]
                n825 = Number To Decimal String(number=w1114) -> (decimal integer string=w1094:string)  [unwired: 1 in]
                n826 = Number To Decimal String(number=w1105) -> (decimal integer string=w1090:string)  [unwired: 1 in]
                n827 = Concatenate Strings("RF Step 9 power" ("string"), w1075, w1075, w1075, ":" ("string"), "\t", w1088, "\r\n") -> (w1096:string)
                n828 = Concatenate Strings("RF Step 10 power" ("string"), w1027, w1027, w1027, ":" ("string"), "\t", w1089, "\r\n") -> (w1095:string)
                n829 = Concatenate Strings("RF Step 7 power" ("string"), w1065, w1065, w1065, ":" ("string"), "\t", w1086, "\r\n") -> (w1098:string)
                n830 = Concatenate Strings("RF Step 8 power" ("string"), w1070, w1070, w1070, ":" ("string"), "\t", w1087, "\r\n") -> (w1097:string)
                n831 = Concatenate Strings("RF Step 6 power" ("string"), w1060, w1060, w1060, ":" ("string"), "\t", w1085, "\r\n") -> (w1099:string)
                n832 = Concatenate Strings("RF Step 4 power" ("string"), w1055, w1055, w1055, ":" ("string"), "\t", w1091, "\r\n") -> (w1101:string)
                n833 = Concatenate Strings("RF Step 5 power" ("string"), w1080, w1080, w1080, ":" ("string"), "\t", w1090, "\r\n") -> (w1100:string)
                n834 = Concatenate Strings("RF Step 2 power" ("string"), w1045, w1045, w1045, ":" ("string"), "\t", w1093, "\r\n") -> (w1103:string)
                n835 = Concatenate Strings("RF Step 3 power" ("string"), w1050, w1050, w1050, ":" ("string"), "\t", w1092, "\r\n") -> (w1102:string)
                n836 = Concatenate Strings("RF Step 1 power" ("string"), w1040, w1040, w1040, ":" ("string"), "\t", w1094, "\r\n") -> (w1104:string)
                n837 = Concatenate Strings("RF Power Steps(power-length)" ("string"), w1031, w1031) -> (w1030:string)
                n838 = Concatenate Strings(w1104, w1103, w1102, w1101, w1100) -> (w1029:string)
                n839 = Concatenate Strings(w1099, w1098, w1097, w1096, w1095) -> (w1028:string)
                n840 = local read "rf step watt 19"() -> (w951:dbl)
                n841 = local read "rf step watt 20"() -> (w954:dbl)
                n842 = local read "rf step watt 17"() -> (w952:dbl)
                n843 = local read "rf step watt 18"() -> (w950:dbl)
                n844 = local read "rf step watt 16"() -> (w953:dbl)
                n845 = local read "rf step watt 14"() -> (w948:dbl)
                n846 = local read "rf step watt 12"() -> (w947:dbl)
                n847 = local read "rf step watt 13"() -> (w949:dbl)
                n848 = local read "rf step watt 11"() -> (w946:dbl)
                n849 = local read "rf step watt 15"() -> (w955:dbl)
                n850 = Number To Decimal String(number=w951) -> (decimal integer string=w972:string)  [unwired: 1 in]
                n851 = Number To Decimal String(number=w954) -> (decimal integer string=w971:string)  [unwired: 1 in]
                n852 = Number To Decimal String(number=w952) -> (decimal integer string=w974:string)  [unwired: 1 in]
                n853 = Number To Decimal String(number=w950) -> (decimal integer string=w973:string)  [unwired: 1 in]
                n854 = Number To Decimal String(number=w953) -> (decimal integer string=w975:string)  [unwired: 1 in]
                n855 = Number To Decimal String(number=w948) -> (decimal integer string=w969:string)  [unwired: 1 in]
                n856 = Number To Decimal String(number=w947) -> (decimal integer string=w967:string)  [unwired: 1 in]
                n857 = Number To Decimal String(number=w949) -> (decimal integer string=w968:string)  [unwired: 1 in]
                n858 = Number To Decimal String(number=w946) -> (decimal integer string=w966:string)  [unwired: 1 in]
                n859 = Number To Decimal String(number=w955) -> (decimal integer string=w970:string)  [unwired: 1 in]
                n860 = Concatenate Strings("RF Step 19 power" ("string"), w985, w985, w985, ":" ("string"), "\t", w972, "\r\n") -> (w964:string)
                n861 = Concatenate Strings("RF Step 20 power" ("string"), w1024, w1024, w1024, ":" ("string"), "\t", w971, "\r\n") -> (w965:string)
                n862 = Concatenate Strings("RF Step 17 power" ("string"), w995, w995, w995, ":" ("string"), "\t", w974, "\r\n") -> (w962:string)
                n863 = Concatenate Strings("RF Step 18 power" ("string"), w990, w990, w990, ":" ("string"), "\t", w973, "\r\n") -> (w963:string)
                n864 = Concatenate Strings("RF Step 16 power" ("string"), w1000, w1000, w1000, ":" ("string"), "\t", w975, "\r\n") -> (w961:string)
                n865 = Concatenate Strings("RF Step 14 power" ("string"), w1005, w1005, w1005, ":" ("string"), "\t", w969, "\r\n") -> (w959:string)
                n866 = Concatenate Strings("RF Step 15 power" ("string"), w980, w980, w980, ":" ("string"), "\t", w970, "\r\n") -> (w960:string)
                n867 = Concatenate Strings("RF Step 12 power" ("string"), w1015, w1015, w1015, ":" ("string"), "\t", w967, "\r\n") -> (w957:string)
                n868 = Concatenate Strings("RF Step 13 power" ("string"), w1010, w1010, w1010, ":" ("string"), "\t", w968, "\r\n") -> (w958:string)
                n869 = Concatenate Strings("RF Step 11 power" ("string"), w1020, w1020, w1020, ":" ("string"), "\t", w966, "\r\n") -> (w956:string)
                n870 = Concatenate Strings(w956, w957, w958, w959, w960) -> (w945:string)
                n871 = Concatenate Strings(w961, w962, w963, w964, w965) -> (w944:string)
                n872 = Concatenate Strings(w1033, w1033, w1030, w1029, w1028, w945, w944) -> (w1034:string)
                n873 = Concatenate Strings(w1036, w1034) -> (w1035:string)
              }
              frame #5 {
                w1179 = "\t"
                w1189 = "\t"
                w1182 = "\t"
                w1184 = "\t"
                w1185 = "\t"
                w1187 = "\t"
                w1192 = "\t"
                w1194 = "\t"
                w1196 = "\t"
                w1197 = "\t"
                w1204 = "\t"
                w1211 = "\r\n"
                w1215 = "\t"
                w1221 = "\r\n"
                w1224 = "\t"
                w1233 = "\t"
                w1258 = "\r\n"
                w1254 = "\t"
                w1244 = "\t"
                w1251 = "\t"
                w1249 = "\t"
                w1248 = "\t"
                w1246 = "\t"
                w1241 = "\t"
                w1239 = "\t"
                w1237 = "\t"
                w1236 = "\t"
                n874 = local read "rf step length 10"() -> (w1302:dbl)
                n875 = local read "rf step length 9"() -> (w1309:dbl)
                n876 = local read "rf step length 7"() -> (w1306:dbl)
                n877 = local read "Pressure set mbar"() -> (w1218:dbl)
                n878 = local read "rf step length 8"() -> (w1310:dbl)
                n879 = local read "rf step length 6"() -> (w1305:dbl)
                n880 = local read "Step Number DC"() -> (w1202:u16)
                n881 = local read "rf step length 4"() -> (w1314:dbl)
                n882 = local read "rf step length 2"() -> (w1317:dbl)
                n883 = local read "rf step length 3"() -> (w1313:dbl)
                n884 = local read "rf step length 1"() -> (w1318:dbl)
                n885 = local read "rf step length 5"() -> (w1301:dbl)
                n886 = local read "Step Number RF"() -> (w1209:u16)
                n887 = local read "Ar set sccm"() -> (w1228:dbl)
                n888 = Number To Decimal String(number=w1309) -> (decimal integer string=w1266:string)  [unwired: 1 in]
                n889 = Number To Decimal String(number=w1302) -> (decimal integer string=w1268:string)  [unwired: 1 in]
                n890 = Number To Decimal String(number=w1306) -> (decimal integer string=w1262:string)  [unwired: 1 in]
                n891 = Number To Decimal String(number=w1310) -> (decimal integer string=w1264:string)  [unwired: 1 in]
                n892 = Number To Decimal String(number=w1305) -> (decimal integer string=w1260:string)  [unwired: 1 in]
                n893 = Number To Decimal String(number=w1314) -> (decimal integer string=w1272:string)  [unwired: 1 in]
                n894 = Number To Decimal String(number=w1317) -> (decimal integer string=w1276:string)  [unwired: 1 in]
                n895 = Number To Decimal String(number=w1313) -> (decimal integer string=w1274:string)  [unwired: 1 in]
                n896 = Number To Decimal String(number=w1318) -> (decimal integer string=w1278:string)  [unwired: 1 in]
                n897 = Number To Decimal String(number=w1202) -> (decimal integer string=w1201:string)  [unwired: 1 in]
                n898 = Number To Decimal String(number=w1301) -> (decimal integer string=w1270:string)  [unwired: 1 in]
                n899 = Number To Decimal String(number=w1228) -> (decimal integer string=w1232:string)  [unwired: 1 in]
                n900 = Format Into String(format string="%.;%f", w1218) -> (resulting string=w1217:string)  [unwired: 2 in, 1 out]
                n901 = Number To Decimal String(number=w1209) -> (decimal integer string=w1208:string)  [unwired: 1 in]
                n902 = Concatenate Strings("RF Step 9 length" ("string"), w1251, w1251, w1251, ":" ("string"), "\t", w1266, "\r\n") -> (w1291:string)
                n903 = Concatenate Strings("RF Step 10 length" ("string"), w1254, w1254, w1254, ":" ("string"), "\t", w1268, "\r\n") -> (w1290:string)
                n904 = Concatenate Strings("RF Step 7 length" ("string"), w1248, w1248, w1248, ":" ("string"), "\t", w1262, "\r\n") -> (w1293:string)
                n905 = Concatenate Strings("RF Step 8 length" ("string"), w1249, w1249, w1249, ":" ("string"), "\t", w1264, "\r\n") -> (w1292:string)
                n906 = Concatenate Strings("RF Step 6 length" ("string"), w1246, w1246, w1246, ":" ("string"), "\t", w1260, "\r\n") -> (w1294:string)
                n907 = Concatenate Strings("RF Step 4 length" ("string"), w1241, w1241, w1241, ":" ("string"), "\t", w1272, "\r\n") -> (w1296:string)
                n908 = Concatenate Strings("RF Step 5 length" ("string"), w1244, w1244, w1244, ":" ("string"), "\t", w1270, "\r\n") -> (w1295:string)
                n909 = Concatenate Strings("RF Step 2 length" ("string"), w1237, w1237, w1237, ":" ("string"), "\t", w1276, "\r\n") -> (w1298:string)
                n910 = Concatenate Strings("RF Step 3 length" ("string"), w1239, w1239, w1239, ":" ("string"), "\t", w1274, "\r\n") -> (w1297:string)
                n911 = Concatenate Strings("RF Step 1 length" ("string"), w1236, w1236, w1236, ":" ("string"), "\t", w1278, "\r\n") -> (w1299:string)
                n912 = Concatenate Strings("Argon Flow(sccm)" ("string"), w1233, w1233, w1233, ":" ("string"), "\t", w1232, "\r\n") -> (w1222:string)
                n913 = Concatenate Strings("Pressure(mbarr)" ("string"), w1224, w1224, w1224, ":" ("string"), "\t", w1217, "\r\n") -> (w1220:string)
                n914 = Concatenate Strings("RF Step Number " ("string"), w1215, w1215, w1215, ":" ("string"), "\t", w1208, "\r\n") -> (w1210:string)
                n915 = Concatenate Strings("DC Step Number" ("string"), w1204, w1204, w1204, ":" ("string"), "\t", w1201, "\r\n") -> (w1200:string)
                n916 = Concatenate Strings(w1299, w1298, w1297, w1296, w1295) -> (w1259:string)
                n917 = Concatenate Strings(w1294, w1293, w1292, w1291, w1290) -> (w1255:string)
                n918 = Concatenate Strings(w1211, w1211, w1210, w1200) -> (w1199:string)
                n919 = Concatenate Strings(w1221, w1221, w1222, w1220, w1199) -> (w1115:string)
                n920 = local read "rf step length 19"() -> (w1129:dbl)
                n921 = local read "rf step length 20"() -> (w1136:dbl)
                n922 = local read "rf step length 17"() -> (w1132:dbl)
                n923 = local read "rf step length 18"() -> (w1128:dbl)
                n924 = local read "rf step length 16"() -> (w1133:dbl)
                n925 = local read "rf step length 14"() -> (w1124:dbl)
                n926 = local read "rf step length 12"() -> (w1121:dbl)
                n927 = local read "rf step length 13"() -> (w1125:dbl)
                n928 = local read "rf step length 11"() -> (w1120:dbl)
                n929 = local read "rf step length 15"() -> (w1137:dbl)
                n930 = Number To Decimal String(number=w1129) -> (decimal integer string=w1172:string)  [unwired: 1 in]
                n931 = Number To Decimal String(number=w1136) -> (decimal integer string=w1170:string)  [unwired: 1 in]
                n932 = Number To Decimal String(number=w1132) -> (decimal integer string=w1176:string)  [unwired: 1 in]
                n933 = Number To Decimal String(number=w1128) -> (decimal integer string=w1174:string)  [unwired: 1 in]
                n934 = Number To Decimal String(number=w1133) -> (decimal integer string=w1178:string)  [unwired: 1 in]
                n935 = Number To Decimal String(number=w1124) -> (decimal integer string=w1166:string)  [unwired: 1 in]
                n936 = Number To Decimal String(number=w1121) -> (decimal integer string=w1162:string)  [unwired: 1 in]
                n937 = Number To Decimal String(number=w1125) -> (decimal integer string=w1164:string)  [unwired: 1 in]
                n938 = Number To Decimal String(number=w1120) -> (decimal integer string=w1160:string)  [unwired: 1 in]
                n939 = Number To Decimal String(number=w1137) -> (decimal integer string=w1168:string)  [unwired: 1 in]
                n940 = Concatenate Strings("RF Step 19 length" ("string"), w1182, w1182, w1182, ":" ("string"), "\t", w1172, "\r\n") -> (w1147:string)
                n941 = Concatenate Strings("RF Step 20 length" ("string"), w1179, w1179, w1179, ":" ("string"), "\t", w1170, "\r\n") -> (w1148:string)
                n942 = Concatenate Strings("RF Step 17 length" ("string"), w1185, w1185, w1185, ":" ("string"), "\t", w1176, "\r\n") -> (w1145:string)
                n943 = Concatenate Strings("RF Step 18 length" ("string"), w1184, w1184, w1184, ":" ("string"), "\t", w1174, "\r\n") -> (w1146:string)
                n944 = Concatenate Strings("RF Step 16 length" ("string"), w1187, w1187, w1187, ":" ("string"), "\t", w1178, "\r\n") -> (w1144:string)
                n945 = Concatenate Strings("RF Step 14 length" ("string"), w1192, w1192, w1192, ":" ("string"), "\t", w1166, "\r\n") -> (w1142:string)
                n946 = Concatenate Strings("RF Step 15 length" ("string"), w1189, w1189, w1189, ":" ("string"), "\t", w1168, "\r\n") -> (w1143:string)
                n947 = Concatenate Strings("RF Step 12 length" ("string"), w1196, w1196, w1196, ":" ("string"), "\t", w1162, "\r\n") -> (w1140:string)
                n948 = Concatenate Strings("RF Step 13 length" ("string"), w1194, w1194, w1194, ":" ("string"), "\t", w1164, "\r\n") -> (w1141:string)
                n949 = Concatenate Strings("RF Step 11 length" ("string"), w1197, w1197, w1197, ":" ("string"), "\t", w1160, "\r\n") -> (w1139:string)
                n950 = Concatenate Strings(w1139, w1140, w1141, w1142, w1143) -> (w1118:string)
                n951 = Concatenate Strings(w1144, w1145, w1146, w1147, w1148) -> (w1116:string)
                n952 = Concatenate Strings(w1118, w1116, w1115) -> (w1117:string)
                n953 = Concatenate Strings(w1258, w1258, w1259, w1255, w1117) -> (w1320:string)
                n954 = Concatenate Strings(w1257, w1320) -> (w1256:string)
              }
              frame #6 {
                n955 = local read "Recipe Name"() -> (w1326:string)
                n956 = call "File Dialog2"("start path"=path "D:/VK-1701 System Files/Recipe Files", "default name"=w1326) -> ("selected path"=w1324:path, "cancelled"=w1323:bool, "error out"=→"error out":errorcluster)  [unwired: 10 in, 1 out]
                n957 = case shown="True" w1323 {
                  tunnel: w1324 -> [w1336 _]
                  tunnel: [w1336 path "" ("selected path")] -> w1321
                  frame False {
                  }
                  frame True {
                  }
                }
                n958 = case shown="False" w1323 {
                  tunnel: w1322 -> [w1329 _]
                  tunnel: w1321 -> [w1328 _]
                  frame False {
                    n959 = Open/Create/Replace File(file path (use dialog)=w1328, operation (0:open)=T4."replace or create", access (0:read/write)=enum16{"read/write", "read-only", "write-only"}."read/write") -> (refnum out=w1331:refnum<file>, error out=w1330:errorcluster)  [unwired: 3 in, 1 out]
                    n960 = Write to Text File(file (use dialog)=w1331, text=w1329, error in=w1330) -> (refnum out=w1333:refnum<file>, error out=w1332:errorcluster)  [unwired: 1 in, 1 out]
                    n961 = Close File(refnum=w1333, error in=w1332) -> ()  [unwired: 2 out]
                  }
                  frame True {
                  }
                }
                "concatenated string" <- w1322
              }
              frame #7 {
              }
            }
          }
        }
        n962 = Equal?(x="flexmag", y="password") -> (x = y?=w456:bool)
        n963 = Equal?(x="password", y="FLEXMAG") -> (x = y?=w455:bool)
        n964 = Or(x=w456, y=w455) -> (x .or. y?=w457:bool)
        n965 = And(x=w457, y="SHOW") -> (x .and. y?=w460:bool)
        n966 = case shown="True" w460 {
          frame False {
          }
          frame True {
            n967 = property on="hidden tab" class="TabCtl (strict)"("Visible"=TRUE) -> ()  [unwired: 2 in, 2 out]
            n968 = property on="concatenated string" class="Str"("Visible"=TRUE) -> ()  [unwired: 2 in, 2 out]
          }
        }
        n969 = local read "CANCEL"() -> (w464:bool)
        n970 = Or(x=w465, y=w464) -> (x .or. y?=w466:bool)
      }
      n971 = while {
        stop <- w24 stop-if-true
        n972 = local read "CANCEL"() -> (w26:bool)
        n973 = local read "done"() -> (w25:bool)
        n974 = Wait Until Next ms Multiple(millisecond multiple=u32 300) -> ()  [unwired: 1 out]
        n975 = case shown="True" "LOAD" {
          frame False {
          }
          frame True {
            n976 = stacked-sequence {
              frame #0 {
                n977 = call "File Dialog"("start path"=path "D:/VK-1701 System Files/Recipe Files") -> ("selected path"=w192:path, "cancelled"=w191:bool, "error out"=→"error out 2":errorcluster)  [unwired: 11 in, 1 out]
                n978 = case shown="True" w191 {
                  tunnel: [w323 string[][] [] ("all rows")] -> w321
                  tunnel: w192 -> [w322 _]
                  frame False {
                    n979 = call-poly <vilib>:"Read Delimited Spreadsheet.vi"("file path (dialog if empty)"=w322) -> ("all rows"=w323:string[][])  [unwired: 9 in, 5 out]
                  }
                  frame True {
                  }
                }
                n980 = Index Array(array=w321, index (row) #1=0 ("index (row)"), index (col) #1=4 ("index (row)"), index (row) #2=1 ("index (row)"), index (col) #2=4 ("index (row)"), index (row) #3=4 ("index (row)"), index (col) #3=4 ("index (row)"), index (row) #4=5 ("index (row)"), index (col) #4=4 ("index (row)"), index (row) #5=8 ("index (row)"), index (col) #5=4 ("index (row)"), index (row) #6=9 ("index (row)"), index (col) #6=4 ("index (row)"), index (row) #7=10 ("index (row)"), index (col) #7=4 ("index (row)"), index (row) #8=13 ("index (row)"), index (col) #8=4 ("index (row)"), index (row) #9=14 ("index (row)"), index (col) #9=4 ("index (row)"), index (row) #10=17 ("index (row)"), index (col) #10=4 ("index (row)"), index (row) #11=18 ("index (row)"), index (col) #11=4 ("index (row)"), index (row) #12=21 ("index (row)"), index (col) #12=4 ("index (row)"), index (row) #13=28 ("index (row)"), index (col) #13=4 ("index (row)"), index (row) #14=29 ("index (row)"), index (col) #14=4 ("index (row)"), index (row) #15=30 ("index (row)"), index (col) #15=4 ("index (row)"), index (row) #16=31 ("index (row)"), index (col) #16=4 ("index (row)"), index (row) #17=32 ("index (row)"), index (col) #17=4 ("index (row)"), index (row) #18=33 ("index (row)"), index (col) #18=4 ("index (row)"), index (row) #19=34 ("index (row)"), index (col) #19=4 ("index (row)"), index (row) #20=35 ("index (row)"), index (col) #20=4 ("index (row)"), index (row) #21=36 ("index (row)"), index (col) #21=4 ("index (row)"), index (row) #22=37 ("index (row)"), index (col) #22=4 ("index (row)"), index (row) #23=38 ("index (row)"), index (col) #23=4 ("index (row)"), index (row) #24=39 ("index (row)"), index (col) #24=4 ("index (row)"), index (row) #25=40 ("index (row)"), index (col) #25=4 ("index (row)"), index (row) #26=41 ("index (row)"), index (col) #26=4 ("index (row)"), index (row) #27=42 ("index (row)"), index (col) #27=4 ("index (row)"), index (row) #28=43 ("index (row)"), index (col) #28=4 ("index (row)"), index (row) #29=44 ("index (row)"), index (col) #29=4 ("index (row)"), index (row) #30=45 ("index (row)"), index (col) #30=4 ("index (row)"), index (row) #31=46 ("index (row)"), index (col) #31=4 ("index (row)"), index (row) #32=47 ("index (row)"), index (col) #32=4 ("index (row)"), index (row) #33=50 ("index (row)"), index (col) #33=4 ("index (row)"), index (row) #34=51 ("index (row)"), index (col) #34=4 ("index (row)"), index (row) #35=52 ("index (row)"), index (col) #35=4 ("index (row)"), index (row) #36=53 ("index (row)"), index (col) #36=4 ("index (row)"), index (row) #37=54 ("index (row)"), index (col) #37=4 ("index (row)"), index (row) #38=55 ("index (row)"), index (col) #38=4 ("index (row)"), index (row) #39=56 ("index (row)"), index (col) #39=4 ("index (row)"), index (row) #40=57 ("index (row)"), index (col) #40=4 ("index (row)"), index (row) #41=58 ("index (row)"), index (col) #41=4 ("index (row)"), index (row) #42=59 ("index (row)"), index (col) #42=4 ("index (row)"), index (row) #43=60 ("index (row)"), index (col) #43=4 ("index (row)"), index (row) #44=61 ("index (row)"), index (col) #44=4 ("index (row)"), index (row) #45=62 ("index (row)"), index (col) #45=4 ("index (row)"), index (row) #46=63 ("index (row)"), index (col) #46=4 ("index (row)"), index (row) #47=64 ("index (row)"), index (col) #47=4 ("index (row)"), index (row) #48=65 ("index (row)"), index (col) #48=4 ("index (row)"), index (row) #49=66 ("index (row)"), index (col) #49=4 ("index (row)"), index (row) #50=67 ("index (row)"), index (col) #50=4 ("index (row)"), index (row) #51=68 ("index (row)"), index (col) #51=4 ("index (row)"), index (row) #52=69 ("index (row)"), index (col) #52=4 ("index (row)"), index (row) #53=74 ("index (row)"), index (col) #53=4 ("index (row)"), index (row) #54=75 ("index (row)"), index (col) #54=4 ("index (row)"), index (row) #55=76 ("index (row)"), index (col) #55=4 ("index (row)"), index (row) #56=77 ("index (row)"), index (col) #56=4 ("index (row)"), index (row) #57=78 ("index (row)"), index (col) #57=4 ("index (row)"), index (row) #58=79 ("index (row)"), index (col) #58=4 ("index (row)"), index (row) #59=80 ("index (row)"), index (col) #59=4 ("index (row)"), index (row) #60=81 ("index (row)"), index (col) #60=4 ("index (row)"), index (row) #61=82 ("index (row)"), index (col) #61=4 ("index (row)"), index (row) #62=83 ("index (row)"), index (col) #62=4 ("index (row)"), index (row) #63=84 ("index (row)"), index (col) #63=4 ("index (row)"), index (row) #64=85 ("index (row)"), index (col) #64=4 ("index (row)"), index (row) #65=86 ("index (row)"), index (col) #65=4 ("index (row)"), index (row) #66=87 ("index (row)"), index (col) #66=4 ("index (row)"), index (row) #67=88 ("index (row)"), index (col) #67=4 ("index (row)"), index (row) #68=89 ("index (row)"), index (col) #68=4 ("index (row)"), index (row) #69=90 ("index (row)"), index (col) #69=4 ("index (row)"), index (row) #70=91 ("index (row)"), index (col) #70=4 ("index (row)"), index (row) #71=92 ("index (row)"), index (col) #71=4 ("index (row)"), index (row) #72=93 ("index (row)"), index (col) #72=4 ("index (row)"), index (row) #73=96 ("index (row)"), index (col) #73=4 ("index (row)"), index (row) #74=97 ("index (row)"), index (col) #74=4 ("index (row)"), index (row) #75=98 ("index (row)"), index (col) #75=4 ("index (row)"), index (row) #76=99 ("index (row)"), index (col) #76=4 ("index (row)"), index (row) #77=100 ("index (row)"), index (col) #77=4 ("index (row)"), index (row) #78=101 ("index (row)"), index (col) #78=4 ("index (row)"), index (row) #79=102 ("index (row)"), index (col) #79=4 ("index (row)"), index (row) #80=103 ("index (row)"), index (col) #80=4 ("index (row)"), index (row) #81=104 ("index (row)"), index (col) #81=4 ("index (row)"), index (row) #82=105 ("index (row)"), index (col) #82=4 ("index (row)"), index (row) #83=106 ("index (row)"), index (col) #83=4 ("index (row)"), index (row) #84=107 ("index (row)"), index (col) #84=4 ("index (row)"), index (row) #85=108 ("index (row)"), index (col) #85=4 ("index (row)"), index (row) #86=109 ("index (row)"), index (col) #86=4 ("index (row)"), index (row) #87=110 ("index (row)"), index (col) #87=4 ("index (row)"), index (row) #88=111 ("index (row)"), index (col) #88=4 ("index (row)"), index (row) #89=112 ("index (row)"), index (col) #89=4 ("index (row)"), index (row) #90=113 ("index (row)"), index (col) #90=4 ("index (row)"), index (row) #91=114 ("index (row)"), index (col) #91=4 ("index (row)"), index (row) #92=115 ("index (row)"), index (col) #92=4 ("index (row)"), index (row) #93=118 ("index (row)"), index (col) #93=4 ("index (row)"), index (row) #94=119 ("index (row)"), index (col) #94=4 ("index (row)"), index (row) #95=122 ("index (row)"), index (col) #95=4 ("index (row)"), index (row) #96=123 ("index (row)"), index (col) #96=4 ("index (row)")) -> (element #1=→"L recipe name":string, element #2=→"L sbs name":string, element #3=→"L recipe selection":string, element #4=→"L web selection":string, element #5=→"L core diamater":string, element #6=→"L left init diamater":string, element #7=→"L web thickness":string, element #8=→"L web speed":string, element #9=→"L tension  value":string, element #10=→"L single process type selection":string, element #11=→"L chamber selection":string, element #12=→"L microwave power":string, element #13=→"L dc power step 1":string, element #14=→"L dc power step 2":string, element #15=→"L dc power step 3":string, element #16=→"L dc power step 4":string, element #17=→"L dc power step 5":string, element #18=→"L dc power step 6":string, element #19=→"L dc power step 7":string, element #20=→"L dc power step 8":string, element #21=→"L dc power step 9":string, element #22=→"L dc power step 10":string, element #23=→"L dc power step 11":string, element #24=→"L dc power step 12":string, element #25=→"L dc power step 13":string, element #26=→"L dc power step 14":string, element #27=→"L dc power step 15":string, element #28=→"L dc power step 16":string, element #29=→"L dc power step 17":string, element #30=→"L dc power step 18":string, element #31=→"L dc power step 19":string, element #32=→"L dc power step 20":string, element #33=→"L dc length step 1":string, element #34=→"L dc length step 2":string, element #35=→"L dc length step 3":string, element #36=→"L dc length step 4":string, element #37=→"L dc length step 5":string, element #38=→"L dc length step 6":string, element #39=→"L dc length step 7":string, element #40=→"L dc length step 8":string, element #41=→"L dc length step 9":string, element #42=→"L dc length step 10":string, element #43=→"L dc length step 11":string, element #44=→"L dc length step 12":string, element #45=→"L dc length step 13":string, element #46=→"L dc length step 14":string, element #47=→"L dc length step 15":string, element #48=→"L dc length step 16":string, element #49=→"L dc length step 17":string, element #50=→"L dc length step 18":string, element #51=→"L dc length step 19":string, element #52=→"L dc length step 20":string, element #53=→"L rf power step 1":string, element #54=→"L rf power step 2":string, element #55=→"L rf power step 3":string, element #56=→"L rf power step 4":string, element #57=→"L rf power step 5":string, element #58=→"L rf power step 6":string, element #59=→"L rf power step 7":string, element #60=→"L rf power step 8":string, element #61=→"L rf power step 9":string, element #62=→"L rf power step 10":string, element #63=→"L rf power step 11":string, element #64=→"L rf power step 12":string, element #65=→"L rf power step 13":string, element #66=→"L rf power step 14":string, element #67=→"L rf power step 15":string, element #68=→"L rf power step 16":string, element #69=→"L rf power step 17":string, element #70=→"L rf power step 18":string, element #71=→"L rf power step 19":string, element #72=→"L rf power step 20":string, element #73=→"L rf length step 1":string, element #74=→"L rf length step 2":string, element #75=→"L rf length step 3":string, element #76=→"L rf length step 4":string, element #77=→"L rf length step 5":string, element #78=→"L rf length step 6":string, element #79=→"L rf length step 7":string, element #80=→"L rf length step 8":string, element #81=→"L rf length step 9":string, element #82=→"L rf length step 10":string, element #83=→"L rf length step 11":string, element #84=→"L rf length step 12":string, element #85=→"L rf length step 13":string, element #86=→"L rf length step 14":string, element #87=→"L rf length step 15":string, element #88=→"L rf length step 16":string, element #89=→"L rf length step 17":string, element #90=→"L rf length step 18":string, element #91=→"L rf length step 19":string, element #92=→"L rf length step 20":string, element #93=→"L argon flow":string, element #94=→"L pressure":string, element #95=→"L rf step number":string, element #96=→"L dc step number":string)
              }
              frame #1 {
                n981 = local read "L dc power step 10"() -> (w394:string)
                n982 = local read "L dc power step 9"() -> (w401:string)
                n983 = local read "L dc power step 8"() -> (w400:string)
                n984 = local read "L dc power step 1"() -> (w418:string)
                n985 = local read "L dc power step 7"() -> (w396:string)
                n986 = local read "L dc power step 2"() -> (w419:string)
                n987 = local read "L dc power step 4"() -> (w404:string)
                n988 = local read "L dc power step 3"() -> (w405:string)
                n989 = local read "L dc power step 5"() -> (w391:string)
                n990 = local read "L dc power step 6"() -> (w397:string)
                n991 = local read "L recipe selection"() -> (w439:string)
                n992 = local read "L web selection"() -> (w435:string)
                n993 = local read "L recipe name"() -> (w441:string)
                n994 = local read "L sbs name"() -> (w440:string)
                n995 = Decimal String To Number(string=w394) -> (number=w393:i32)  [unwired: 2 in, 1 out]
                n996 = Decimal String To Number(string=w401) -> (number=w402:i32)  [unwired: 2 in, 1 out]
                n997 = Decimal String To Number(string=w400) -> (number=w399:i32)  [unwired: 2 in, 1 out]
                n998 = Decimal String To Number(string=w418) -> (number=w417:i32)  [unwired: 2 in, 1 out]
                n999 = Decimal String To Number(string=w396) -> (number=w395:i32)  [unwired: 2 in, 1 out]
                n1000 = Decimal String To Number(string=w419) -> (number=w420:i32)  [unwired: 2 in, 1 out]
                n1001 = Decimal String To Number(string=w404) -> (number=w403:i32)  [unwired: 2 in, 1 out]
                n1002 = Decimal String To Number(string=w405) -> (number=w406:i32)  [unwired: 2 in, 1 out]
                n1003 = Decimal String To Number(string=w391) -> (number=w392:i32)  [unwired: 2 in, 1 out]
                n1004 = Decimal String To Number(string=w397) -> (number=w398:i32)  [unwired: 2 in, 1 out]
                n1005 = Equal?(x=w435, y="Web") -> (x = y?=w433:bool)
                n1006 = Equal?(x=w439, y="Single Recipe") -> (x = y?=w437:bool)
                n1007 = local write "dc step watt 10"(w393) -> ()
                n1008 = local write "dc step watt 9"(w402) -> ()
                n1009 = local write "dc step watt 1"(w417) -> ()
                n1010 = local write "dc step watt 8"(w399) -> ()
                n1011 = local write "dc step watt 7"(w395) -> ()
                n1012 = local write "dc step watt 2"(w420) -> ()
                n1013 = local write "dc step watt 4"(w403) -> ()
                n1014 = local write "dc step watt 3"(w406) -> ()
                n1015 = local write "dc step watt 5"(w392) -> ()
                n1016 = local write "dc step watt 6"(w398) -> ()
                n1017 = case shown="True" w437 {
                  tunnel: [w453 w454] -> w436
                  frame False {
                    w453 = u16 1 items=["single recipe", "multilayer recipe"] ("Recipe Selection")
                  }
                  frame True {
                    w454 = u16 0 items=["single recipe", "multilayer recipe"] ("Recipe Selection")
                  }
                }
                n1018 = case shown="False" w433 {
                  tunnel: [w451 w452] -> w432
                  frame False {
                    w451 = u16 1 items=["web", "other"] ("Web Selection")
                  }
                  frame True {
                    w452 = u16 0 items=["web", "other"] ("Web Selection")
                  }
                }
                n1019 = local write "Substrate Material"(w440) -> ()
                n1020 = local write "Recipe Name"(w441) -> ()
                n1021 = local read "L dc length step 1"() -> (w373:string)
                n1022 = local read "L dc length step 10"() -> (w387:string)
                n1023 = local read "L dc length step 7"() -> (w385:string)
                n1024 = local read "L dc length step 2"() -> (w372:string)
                n1025 = local read "L dc length step 4"() -> (w377:string)
                n1026 = local read "L dc length step 9"() -> (w380:string)
                n1027 = local read "L dc length step 3"() -> (w376:string)
                n1028 = local read "L dc length step 5"() -> (w390:string)
                n1029 = local read "L dc length step 6"() -> (w384:string)
                n1030 = local read "L dc length step 8"() -> (w381:string)
                n1031 = local write "Recipe Selection"(w436) -> ()
                n1032 = local write "Web Selection"(w432) -> ()
                n1033 = Wait (ms)(milliseconds to wait=u32 100) -> ()  [unwired: 1 out]
                n1034 = Decimal String To Number(string=w373) -> (number=w374:i32)  [unwired: 2 in, 1 out]
                n1035 = Decimal String To Number(string=w385) -> (number=w386:i32)  [unwired: 2 in, 1 out]
                n1036 = Decimal String To Number(string=w372) -> (number=w371:i32)  [unwired: 2 in, 1 out]
                n1037 = Decimal String To Number(string=w377) -> (number=w378:i32)  [unwired: 2 in, 1 out]
                n1038 = Decimal String To Number(string=w380) -> (number=w379:i32)  [unwired: 2 in, 1 out]
                n1039 = Decimal String To Number(string=w387) -> (number=w388:i32)  [unwired: 2 in, 1 out]
                n1040 = Decimal String To Number(string=w376) -> (number=w375:i32)  [unwired: 2 in, 1 out]
                n1041 = Decimal String To Number(string=w390) -> (number=w389:i32)  [unwired: 2 in, 1 out]
                n1042 = Decimal String To Number(string=w384) -> (number=w383:i32)  [unwired: 2 in, 1 out]
                n1043 = Decimal String To Number(string=w381) -> (number=w382:i32)  [unwired: 2 in, 1 out]
                n1044 = local write "dc step length 1"(w374) -> ()
                n1045 = local write "dc step length 10"(w388) -> ()
                n1046 = local write "dc step length 7"(w386) -> ()
                n1047 = local write "dc step length 2"(w371) -> ()
                n1048 = local write "dc step length 4"(w378) -> ()
                n1049 = local write "dc step length 9"(w379) -> ()
                n1050 = local write "dc step length 3"(w375) -> ()
                n1051 = local write "dc step length 5"(w389) -> ()
                n1052 = local write "dc step length 6"(w383) -> ()
                n1053 = local write "dc step length 8"(w382) -> ()
                n1054 = local read "L microwave power"() -> (w415:string)
                n1055 = local read "L left init diamater"() -> (w430:string)
                n1056 = local read "L core diamater"() -> (w431:string)
                n1057 = local read "L web thickness"() -> (w425:string)
                n1058 = local read "L tension  value"() -> (w421:string)
                n1059 = local read "L web speed"() -> (w424:string)
                n1060 = Decimal String To Number(string=w415) -> (number=w416:i32)  [unwired: 2 in, 1 out]
                n1061 = Decimal String To Number(string=w431) -> (number=w429:i32)  [unwired: 2 in, 1 out]
                n1062 = Decimal String To Number(string=w425) -> (number=w426:i32)  [unwired: 2 in, 1 out]
                n1063 = Decimal String To Number(string=w421) -> (number=w422:i32)  [unwired: 2 in, 1 out]
                n1064 = Decimal String To Number(string=w424) -> (number=w423:i32)  [unwired: 2 in, 1 out]
                n1065 = Fract/Exp String To Number(use system decimal point (T)=FALSE, string=w430) -> (number=w428:dbl)  [unwired: 2 in, 1 out]
                n1066 = local write "power microwave"(w416) -> ()
                n1067 = local write "left initial diameter"(w428) -> ()
                n1068 = local write "core diameter"(w429) -> ()
                n1069 = local write "web thickness"(w426) -> ()
                n1070 = local write "tension value"(w422) -> ()
                n1071 = local write "web speed"(w423) -> ()
                n1072 = local read "L rf power step 10"() -> (w347:string)
                n1073 = local read "L rf power step 9"() -> (w340:string)
                n1074 = local read "L rf power step 8"() -> (w341:string)
                n1075 = local read "L rf power step 1"() -> (w333:string)
                n1076 = local read "L rf power step 7"() -> (w345:string)
                n1077 = local read "L dc power step 6"() -> (w344:string)
                n1078 = local read "L rf power step 2"() -> (w332:string)
                n1079 = local read "L rf power step 4"() -> (w337:string)
                n1080 = local read "L rf power step 3"() -> (w336:string)
                n1081 = local read "L rf power step 5"() -> (w350:string)
                n1082 = Decimal String To Number(string=w347) -> (number=w348:i32)  [unwired: 2 in, 1 out]
                n1083 = local read "L single process type selection"() -> (w414:string)
                n1084 = Decimal String To Number(string=w340) -> (number=w339:i32)  [unwired: 2 in, 1 out]
                n1085 = Decimal String To Number(string=w341) -> (number=w342:i32)  [unwired: 2 in, 1 out]
                n1086 = Decimal String To Number(string=w333) -> (number=w334:i32)  [unwired: 2 in, 1 out]
                n1087 = Decimal String To Number(string=w345) -> (number=w346:i32)  [unwired: 2 in, 1 out]
                n1088 = Decimal String To Number(string=w332) -> (number=w331:i32)  [unwired: 2 in, 1 out]
                n1089 = Decimal String To Number(string=w337) -> (number=w338:i32)  [unwired: 2 in, 1 out]
                n1090 = Decimal String To Number(string=w336) -> (number=w335:i32)  [unwired: 2 in, 1 out]
                n1091 = Decimal String To Number(string=w350) -> (number=w349:i32)  [unwired: 2 in, 1 out]
                n1092 = Decimal String To Number(string=w344) -> (number=w343:i32)  [unwired: 2 in, 1 out]
                n1093 = local read "L chamber selection"() -> (w410:string)
                n1094 = local write "rf step watt 10"(w348) -> ()
                n1095 = local write "rf step watt 9"(w339) -> ()
                n1096 = local write "rf step watt 8"(w342) -> ()
                n1097 = local write "rf step watt 1"(w334) -> ()
                n1098 = local write "rf step watt 7"(w346) -> ()
                n1099 = local write "rf step watt 2"(w331) -> ()
                n1100 = local write "rf step watt 4"(w338) -> ()
                n1101 = local write "rf step watt 3"(w335) -> ()
                n1102 = local write "rf step watt 5"(w349) -> ()
                n1103 = local write "rf step watt 6"(w343) -> ()
                n1104 = Equal?(x=w410, y="III" ("L single process")) -> (x = y?=w408:bool)
                n1105 = Equal?(x=w414, y="Microwave" ("L single process")) -> (x = y?=w412:bool)
                n1106 = case shown="True" w412 {
                  tunnel: [w444 enum32{"microwave", "dcsputter", "rfsputter"}."microwave" ("single process selection")] -> w411
                  frame False {
                    n1107 = local read "L single process type selection"() -> (w446:string)
                    n1108 = Equal?(x=w446, y="RF Sputter" ("L single process")) -> (x = y?=w445:bool)
                    n1109 = case shown="False" w445 {
                      tunnel: [enum32{"microwave", "dcsputter", "rfsputter"}."dcsputter" ("single process selection") enum32{"microwave", "dcsputter", "rfsputter"}."rfsputter" ("single process selection")] -> w444
                      frame False {
                      }
                      frame True {
                      }
                    }
                  }
                  frame True {
                  }
                }
                n1110 = case shown="False" w408 {
                  tunnel: [enum32{"chamber II", "chamber III"}."chamber II" ("DC Sputter Chamber Selection") enum32{"chamber II", "chamber III"}."chamber III" ("DC Sputter Chamber Selection")] -> w407
                  frame False {
                  }
                  frame True {
                  }
                }
                n1111 = local read "L pressure"() -> (w327:string)
                n1112 = local read "L rf length step 1"() -> (w368:string)
                n1113 = local read "L rf length step 10"() -> (w354:string)
                n1114 = local read "L argon flow"() -> (w325:string)
                n1115 = local read "L rf length step 7"() -> (w356:string)
                n1116 = local read "L rf length step 2"() -> (w369:string)
                n1117 = local read "L rf length step 4"() -> (w364:string)
                n1118 = local read "L rf length step 9"() -> (w361:string)
                n1119 = local read "L rf length step 3"() -> (w365:string)
                n1120 = local read "L rf length step 5"() -> (w351:string)
                n1121 = local read "L rf length step 6"() -> (w357:string)
                n1122 = local read "L rf length step 8"() -> (w360:string)
                n1123 = Fract/Exp String To Number(use system decimal point (T)=FALSE, string=w327) -> (number=w328:dbl)  [unwired: 2 in, 1 out]
                n1124 = Decimal String To Number(string=w325) -> (number=w326:i32)  [unwired: 2 in, 1 out]
                n1125 = Decimal String To Number(string=w368) -> (number=w367:i32)  [unwired: 2 in, 1 out]
                n1126 = Decimal String To Number(string=w356) -> (number=w355:i32)  [unwired: 2 in, 1 out]
                n1127 = Decimal String To Number(string=w369) -> (number=w370:i32)  [unwired: 2 in, 1 out]
                n1128 = Decimal String To Number(string=w364) -> (number=w363:i32)  [unwired: 2 in, 1 out]
                n1129 = Decimal String To Number(string=w361) -> (number=w362:i32)  [unwired: 2 in, 1 out]
                n1130 = Decimal String To Number(string=w354) -> (number=w353:i32)  [unwired: 2 in, 1 out]
                n1131 = Decimal String To Number(string=w365) -> (number=w366:i32)  [unwired: 2 in, 1 out]
                n1132 = Decimal String To Number(string=w351) -> (number=w352:i32)  [unwired: 2 in, 1 out]
                n1133 = Decimal String To Number(string=w357) -> (number=w358:i32)  [unwired: 2 in, 1 out]
                n1134 = Decimal String To Number(string=w360) -> (number=w359:i32)  [unwired: 2 in, 1 out]
                n1135 = local write "DC Sputter Chamber Selection"(w407) -> ()
                n1136 = local write "Pressure set mbar"(w328) -> ()
                n1137 = local write "Ar set sccm"(w326) -> ()
                n1138 = local write "rf step length 1"(w367) -> ()
                n1139 = local write "rf step length 10"(w353) -> ()
                n1140 = local write "rf step length 7"(w355) -> ()
                n1141 = local write "rf step length 2"(w370) -> ()
                n1142 = local write "rf step length 4"(w363) -> ()
                n1143 = local write "rf step length 9"(w362) -> ()
                n1144 = local write "rf step length 3"(w366) -> ()
                n1145 = local write "rf step length 5"(w352) -> ()
                n1146 = local write "rf step length 6"(w358) -> ()
                n1147 = local write "rf step length 8"(w359) -> ()
                n1148 = local write "single process selection"(w411) -> ()
              }
            }
          }
        }
        n1149 = Or(x=w25, y=w26) -> (x .or. y?=w24:bool)
      }
    }
  }
